vi "CRYAcquisition Editor.vi"() -> ()   [LabVIEW 2013]
uses:
  <vilib>/Utility/miscctls.llb/LVBoundsTypeDef.ctl
  Typedef Control/CRYAcquisition Cluster.ctl
  Typedef Control/CRYHardware Channel Info.ctl
  Typedef Control/CRYWaveform Cluster.ctl
  Typedef Control/CRYData Cluster.ctl
  CRYMainGlobal.vi
  CRYProject/CRYProject Editor Global.vi
  CRYWindow/SubVI/CRYMain Sub Window Global.vi
  Misc/SubVI/CRYMisc vis settings global.vi
  CRYStepSetup/CRYStepSetup Global.vi
panel:
  out "Acquisition Bk":T1={"Mode"=1, "Name"="", "use ch name"=FALSE, "Record Time"=10.0, "hide rec"=FALSE, "hide play"=FALSE, "rec delay"=0.0, "rec pad"=0.0, "dcc units"=0, "sine gen setting"="", "scope_fft setting"="", "voltmeter setting"="", "rta setting"="", "trig offset(sec)"=0.0, "triggered  record"=FALSE, "trig level"=0.0, "trig unit"=0, "trig slop"=FALSE, "trig timeout(sec)"=0.0, "add record"=FALSE, "EQ"=FALSE, "record table"=[], "play table"=[], "trig channel"="", "Help"=""} {"trig timeout(sec)" format="%.2f"; "trig level" format="%.2f"; "trig offset(sec)" format="%.2f"; "rec delay" format="%.2f"; "rec pad" format="%.2f"; "Record Time" format="%.2f"}
  out "Origin MR0":string[][](array[string])
  in  "Channels Change?":bool
  in  "Change Record Name?":bool
  out "Old MR0":string[][](array[string])
  out "Changed Curve":string[][](array[string])
  in  "AddStep":bool
  in  "Add Lib":bool
  in  "Board Tab":enum32{"Page 1"}(tab)
  in  "Cancel":bool caption="Apply"
  in  "OK":bool caption="Apply"
  in  "Sub Board Tab":enum32{"Setting", "Help"}(tab)
  in  "Mode Tab":T2(tab)
  out "Record0":bool caption="采集"
  in  "WFMRing":u16(ring) items=["Stimulus"]
  in  "MP0":i32(listbox)
  in  "O_Channel0":bool
  out "MR0":string[][](table)
  in  "I_Channel0":bool caption="Boolean 2"
  in  "Time R0":dbl caption="预采集时间(秒)" format="%#_6p"
  out "Play0":bool caption="播放"
  out "Trigger Boolean":bool caption="Record Trigger"
  in  "Triger1":bool caption="触发"
  in  "Trigger Level1":dbl caption="触发电平" format="%#.3p"
  in  "Trigger Offset1":dbl caption="触发偏移(s)" format="%#.3p"
  in  "Trigger Channel1":u16(ring) caption="触发通道" items=["Direct In 1", "Direct In 2", "Direct In 3", "Direct In 4", "Mic 1", "Mic 2", "Mic 3", "Mic 4", "DUT Mic L", "DUT Mic Current L", "Imp 1L", "Imp 1R", "LineIn L", "LineIn R", "USB In L", "USB In R"]
  in  "Time Out1":dbl caption="时间结束(s)" format="%#.3p"
  in  "Trigger Unit1_1":bool caption="触发单位"
  in  "Trigger Unit1_2":bool caption="Trigger Unit Pa"
  in  "Slop1+1":bool caption="斜率"
  in  "Slop1-1":bool
  in  "I_Channel1":bool
  in  "Time R1":dbl caption="采集时间(秒)" format="%#_6p"
  in  "MR1":string[][](table)
  out "Record1":bool caption="采集"
  out "Record1_1":bool caption="采集触发"
  in  "Hide P P2":bool caption="隐藏面板"
  in  "Config P2":bool
  out "Play2":bool caption="播放"
  in  "HideP R3":bool caption="隐藏面板"
  in  "Config R3":bool
  in  "MR3":string[][](table)
  out "Record3":bool caption="采集"
  in  "Config R4":bool
  in  "Hide P R4":bool caption="隐藏面板"
  in  "MR4":string[][](table)
  out "Record4":bool caption="采集"
  in  "Config R5":bool
  in  "Hide P R5":bool caption="隐藏面板"
  in  "MR5":string[][](table)
  out "Record5":bool caption="采集"
  in  "Config R6":bool
  in  "Hide P R6":bool caption="隐藏面板"
  in  "Delay R6":dbl caption="采集延迟(秒)" format="%#_6p"
  in  "MR6":string[][](table)
  out "Record6":bool caption="采集"
  in  "Hide P P7":bool caption="隐藏面板"
  in  "Config P7":bool
  in  "Config R7":bool
  in  "Hide P R7":bool caption="隐藏面板"
  in  "Delay R7":dbl caption="采集延迟(秒)" format="%#_6p"
  in  "MR7":string[][](table)
  out "Record7":bool caption="采集"
  out "Play7":bool caption="播放"
  in  "Hide P P8":bool caption="隐藏面板"
  in  "Config P8":bool
  in  "Config R8":bool
  in  "Hide P R8":bool caption="隐藏面板"
  in  "Delay R8":dbl caption="采集延迟(秒)" format="%#_6p"
  in  "MR8":string[][](table)
  out "Record8":bool caption="采集"
  out "Play8":bool caption="播放"
  in  "Hide P P9":bool caption="隐藏面板"
  in  "Config P9":bool
  in  "Config R9":bool
  in  "Hide P R9":bool caption="隐藏面板"
  in  "Delay R9":dbl caption="采集延迟(秒)" format="%#_6p"
  in  "MR9":string[][](table)
  out "Record9":bool caption="采集"
  out "Play9":bool caption="播放"
  in  "Hide P P10":bool caption="隐藏面板"
  in  "Config P10":bool
  in  "Config R10":bool
  in  "Hide P R10":bool caption="隐藏面板"
  in  "Delay R10":dbl caption="采集延迟(秒)" format="%#_6p"
  in  "MR10":string[][](table)
  out "Record10":bool caption="采集"
  out "Play10":bool caption="播放"
  in  "Record11":enum32{"Radio Selection 1", "Radio Selection 2"}(radio) caption="采集"
  out "Discription String":string
  in  "Record Curve Name":string caption="记录曲线名称"
  in  "Use Channel Name":bool=TRUE caption="使用通道名称"
  in  "Mode Select":u16(ring) caption="模式选择" items=["播放和采集", "采集", "信号发生器", "多功能表", "示波器", "频谱分析仪", "实时频谱分析仪", "信号发生器/多功能表", "信号发生器/示波器", "信号发生器/频谱分析仪", "信号发生器/实时频谱分析仪", "读取直流连接"]
  in  "Help":string
  in  "Apply":bool
  in  "Load...":bool caption="Apply"
  in  "Revert":bool caption="Apply"
  in  "Save As...":bool caption="Apply"
  in  "CurveReplace":bool caption="Use Channel Name"
  out "EndFlag":bool
  in  "Curve Change":enum16{"Curves", "Values", "Results", "WFM"}[](array[ring])
  in  "Started":bool
  in  "Execution control":T3={"interactive"=TRUE, "displayed"=TRUE, "in a seq"=FALSE}
  in  "Run flag":bool caption="Use Channel Name"
  out "Selected I_channel Info":T4[](array[typedef]) {"Coupling" items=["Default"=-1, "RSE"=10083, "NRSE"=10078, "Differential"=10106, "Pseudodifferential"=12529]; "term config" items=["Default"=-1, "RSE"=10083, "NRSE"=10078, "Differential"=10106, "Pseudodifferential"=12529]; "Anti-aliasing Factor (%fs)" format="%.2f"}
  out "Selected O_channel Info":T4[](array[typedef]) {"Coupling" items=["Default"=-1, "RSE"=10083, "NRSE"=10078, "Differential"=10106, "Pseudodifferential"=12529]; "term config" items=["Default"=-1, "RSE"=10083, "NRSE"=10078, "Differential"=10106, "Pseudodifferential"=12529]; "Anti-aliasing Factor (%fs)" format="%.2f"}
  in  "Calibration In":string
  in  "Hardware In":string
  in  "stop":bool
  out "Column":i32
  out "Row":i32
  out "I_channel Info":T4[](array[typedef]) caption="I_channel Info Out" {"Coupling" items=["Default"=-1, "RSE"=10083, "NRSE"=10078, "Differential"=10106, "Pseudodifferential"=12529]; "term config" items=["Default"=-1, "RSE"=10083, "NRSE"=10078, "Differential"=10106, "Pseudodifferential"=12529]; "Anti-aliasing Factor (%fs)" format="%.2f"}
  out "O_channel Info":T4[](array[typedef]) {"Coupling" items=["Default"=-1, "RSE"=10083, "NRSE"=10078, "Differential"=10106, "Pseudodifferential"=12529]; "term config" items=["Default"=-1, "RSE"=10083, "NRSE"=10078, "Differential"=10106, "Pseudodifferential"=12529]; "Anti-aliasing Factor (%fs)" format="%.2f"}
  out "Proper VI No":i32
  in  "Load Test":bool
  in  "Acquisition":T1={"Mode"=1, "Name"="", "use ch name"=FALSE, "Record Time"=10.0, "hide rec"=FALSE, "hide play"=FALSE, "rec delay"=0.0, "rec pad"=0.0, "dcc units"=0, "sine gen setting"="", "scope_fft setting"="", "voltmeter setting"="", "rta setting"="", "trig offset(sec)"=0.0, "triggered  record"=FALSE, "trig level"=0.0, "trig unit"=0, "trig slop"=FALSE, "trig timeout(sec)"=0.0, "add record"=FALSE, "EQ"=FALSE, "record table"=[], "play table"=[], "trig channel"="", "Help"=""} {"trig timeout(sec)" format="%.2f"; "trig level" format="%.2f"; "trig offset(sec)" format="%.2f"; "rec delay" format="%.2f"; "rec pad" format="%.2f"; "Record Time" format="%.2f"}
  out "VIMiniumBound":T5
  # "dB"
  # "+"
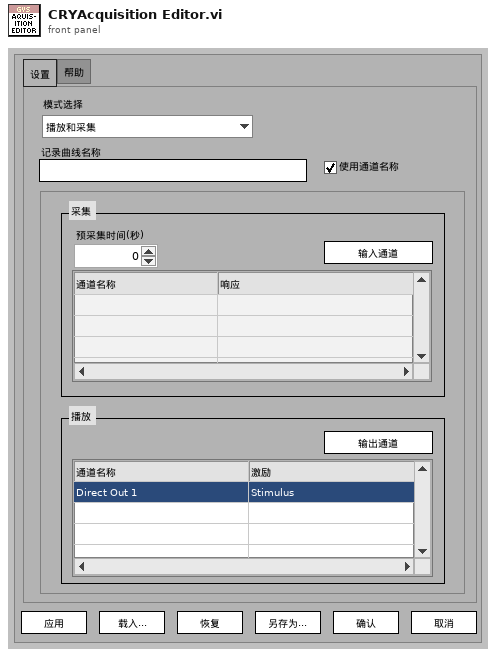
[diagram p1: front panel]
types:
  T1 = typedef "CRYAcquisition Cluster.ctl" = cluster{"Mode":u16, "Name":string, "use ch name":bool, "Record Time":dbl, "hide rec":bool, "hide play":bool, "rec delay":dbl, "rec pad":dbl, "dcc units":i8, "sine gen setting":string, "scope_fft setting":string, "voltmeter setting":string, "rta setting":string, "trig offset(sec)":dbl, "triggered  record":bool, "trig level":dbl, "trig unit":u8, "trig slop":bool, "trig timeout(sec)":dbl, "add record":bool, "EQ":bool, "record table":string[][], "play table":string[][], "trig channel":string, "Help":string}
  T2 = enum32{"0", "1", "2", "3", "4", "5", "6", "7", "8", "9", "10", "11"}
  T3 = cluster{"interactive":bool, "displayed":bool, "in a seq":bool}
  T4 = typedef "CRYHardware Channel Info.ctl" = cluster{"ID":i32, "Name":string, "Digital":bool, "Input":bool, "Device Name":string, "Hardware Ch ID":u8, "Vmax (V)":dbl, "Latency (samples)":dbl, "Sampling Rate (Hz)":u32, "Bit Depth":u32, "Anti-aliasing Factor (%fs)":sgl, "DAQmx Channel":tag, "term config":i32, "Coupling":i32, "IEPE en":bool, "ASIOChannel Name":string, "Audio Driver":u16, "ASIOChannel Index":u8}
  T5 = typedef "LVBoundsTypeDef.ctl" = cluster{"Width":u32, "Height":u32}
  T6 = typedef "CRYData Cluster.ctl" = cluster{"Name":string, "Curve":cluster{"x":dbl, "y":dbl, "z":dbl}[], "X data":u16, "Y data":u16, "Z data":u16, "X axis":u16, "Y axis":u16, "Z axis":u16, "X unit":string, "Y unit":string, "Z unit":string, "X dB ref":dbl, "Y dB ref":dbl, "Z dB ref":dbl, "single val":bool, "protected":bool, "display X":bool, "display Y":bool, "display Z":bool, "Test Info":string, "Step No.":i32, "Plot Settings":cluster{"Color":u32, "Interpolation":u8, "Point Style":u8, "Line Style":u8, "Point Color":u32, "Line Width":u8, "Bar Plot Style":u8, "Fill To":i16}, "AutoProtect":bool}
  T7 = typedef "CRYWaveform Cluster.ctl" = cluster{"Waveform":cluster{"X0":dbl, "dX":dbl, "Y":sgl[]}, "X data":u16, "Y data":u16, "Y axis":u16, "X unit":string, "Y unit":string, "Y dB ref":dbl, "display Y":bool, "display X":bool, "Overload?":bool, "Test Info":string, "Step No.":i32, "Name":string, "protected":bool, "Sqc history":string[], "Signal Channel ID":i32, "Plot Settings":cluster{"Color":u32, "Interpolation":u8, "Point Style":u8, "Line Style":u8, "Point Color":u32, "Line Width":u8, "Bar Plot Style":u8, "Fill To":i16}, "AutoProtect":bool}
  T8 = typedef "CRYStep.ctl" = cluster{"No.VI":i32, "Category":string, "StepName":string, "Seq setup flattened":string, "Comment":string, "Steps config.":bool[], "Jump config":i32[], "Start":dbl, "Increment":dbl, "Name":string, "Unit":string, "Y data":u16, "Y prefix":string, "Y dB ref":dbl, "Y unit":string, "Repeat State Array":cluster{"Start":dbl, "Increment":dbl, "Count":i32, "Num":i32}[]}
  T9 = enum16{"OK", "Yes", "YesNo", "YesNoCancel", "ReplaceAppend"}
  T10 = typedef "LVPoint32TypeDef.ctl" = cluster{"Horizontal":i32, "Vertical":i32}
  T11 = typedef "LVRowAndColumnTypeDef.ctl" = cluster{"Row":i32, "Column":i32}
  T12 = typedef "LVPositionTypeDef.ctl" = cluster{"Left":i32, "Top":i32}
  T13 = typedef "CRYWaveform Cluster Array.ctl" = T7[]
  T14 = typedef "CRYCalibration 2DCluster.ctl" = cluster{"Calibration":T15, "Corr Curve":T6, "EQ Curve":T6, "Sens Curve":T6}
  T15 = typedef "CRYCalibration Cluster.ctl" = cluster{"Calibration Step Name":string, "Device":string, "Correction Curve Name":string, "Equalization Curve Name":string, "Sensitivity Curve Name":string, "Corr Folder and File":string, "EQ Folder and File":string, "Sens Folder and File":string, "Corr Step size":u16, "EQ Step size":u16, "Input":bool, "Last Cal Date (sec)":timestamp, "Cha Name":string, "Corr Curve Found":bool, "EQ Curve Found":bool, "Sens Curve Found":bool, "Signal Type":string, "Calibrated Device":string, "Hz":u32}
  T16 = cluster{"Load Test":bool, "I_Channel0":bool, "O_Channel0":bool, "I_Channel1":bool, "Config P2":bool, "Config R3":bool, "Config R4":bool, "Config R5":bool, "Config R6":bool, "Config R7":bool, "Config P7":bool, "Config R8":bool, "Config P8":bool, "Config R9":bool, "Config P9":bool, "Config R10":bool, "Config P10":bool, "Add Lib":bool, "OK":bool, "Cancel":bool}
  T17 = typedef "CRYCalibration All Cluster.ctl" = cluster{"Calibration 2D":T14[], "Help":string, "Tab Value":i32, "Input Signal Type":string, "Output Signal Type":string}
  T18 = typedef "CRYHardware.ctl" = cluster{"Name":string, "Analog I/O":u16, "Digital I/O":u16, "Channels":u8, "Dig Dev ID":u8, "N ports":u8, "Interface":u32, "Dig I/O Ports":cluster{"port #":i16, "width":i16, "direction":i32}[], "Interf settings":cluster{"Type":u16, "COM Port":u8, "Baud rate":u32, "Data bits":u32, "Parity":u16, "Stop bits":u16, "Flow control":u16, "Dev ID IEEE":u8}[], "N interfs":i32, "udev SNs":i16[], "udev enable":bool, "Channel Array":T4[], "Cal sequence":string, "SelectedIn":u16, "SelectedOut":u16, "SelectedTab":u16, "State":bool, "Help":string, "Advanced":bool, "In Audio Driver":u16, "Out Audio Driver":u16}
  T19 = cluster{"StepName":string, "setup flattened":string}[]
  T20 = cluster{"StepName":string, "setup flattened":string}
  T21 = typedef "CRYStimulus Cluster.ctl" = cluster{"StimulusType":string, "UseMLValArray":u16[], "ML_axisArray":u16[], "MLValLevelNameArray":string[], "Level(U)Array":dbl[], "Start(Stop)FreqArray":dbl[], "Start(Stop)AmpArray":dbl[], "StepResolutionArray":u16[], "Unit_Array":u16[], "DegValArray":dbl[], "DegUnitArray":string[], "Steps1":i32, "Cycle/step1(#)":u32, "Time/step1(s)":dbl, "Transition1":dbl, "SweepRate2":dbl, "Freq3(Hz)":dbl, "Steps3(#)":dbl, "Cycles3(#)":u32, "StepSize3":dbl, "wave time":string, "RMS_Value4":dbl, "Peak_Value4":dbl, "WavePath4":string, "RMS_unit4":string, "Peak_unit4":string, "wave Info":string, "dc_ctrl5_1":u16, "dc_ctrl5_2":u16, "dc_polar5":u16, "Max.Current":u16, "Steps5(#)":u32, "Time/Step5":dbl, "Level5":dbl, "StepsSize5Val":dbl, "StepSize5Unit":string, "SweepType":u16, "Fixed/Ratio6":u16, "Transition6":dbl, "Steps6(#)":dbl, "Cycle/Steps6(#)":u32, "Time/Steps6(s)":dbl, "Freq6(Hz)":dbl, "Difference6(Hz)":dbl, "Ratio6":string, "NoiseType7":u16, "Duration7(s)":dbl, "MinFreq7(Hz)":dbl, "MaxFreq7(Hz)":dbl, "MinFreq8(Hz)":dbl, "MaxFreq8(Hz)":dbl, "FreqRounding8":bool, "Duration8(s)":dbl, "Tones8":dbl, "RoundingVal8":dbl, "ApplyEQ":bool, "Duration(s)":dbl, "CustomStimulusName ":string, "Flatten Element Array":string[], "sine waves":cluster{"freq":dbl, "ampl":dbl, "cycles":dbl}[], "Channel Out":i32, "RatioVal6":dbl, "TabCtrl6":enum32{"Master Tone", "Slave Tone"}, "Signal Type Name":string, "Help":string, "Channel Sel":u16, "V on DUT":bool, "Output Imp":dbl, "Nominal Imp":dbl}
  T22 = cluster{"Signal Type":string, "CustomStimulusName ":string}
  T23 = cluster{"gen'r mode":i32, "frequency":u32, "output level":dbl, "wave path":string, "wav play mode":i32, "duration":dbl, "n times":i32, "channel":i32, "wav level":dbl, "EQ":bool, "f knob log":bool, "f knob low":dbl, "f knob high":dbl, "ol knob log":bool, "ol knob low":dbl, "ol knob high":dbl, "Lin Display Prefs":string, "dB Display Prefs":string, "Duration noise":dbl, "Min freq noise":dbl, "Max freq noise":dbl, "Channel String":string, "Play Sine Wave":i32}
  T24 = typedef "CRYMultimeter.ctl" = cluster{"Ave/Max/Min":i32, "Level":i32, "Channel":i32, "Signal Type":string, "Weighting":string, "Applay Correction":bool, "lin/exp avg":u16, "rec time (sec)":dbl, "Average Time (Sec)":dbl, "Lin Display Prefs":string, "dB Display Prefs":string, "Time Weighting":u16, "Display":u16}
  T25 = typedef "CRYScope-FFT.ctl" = cluster{"window":i32, "n avgs":i32, "lin/exp avg":i32, "pwr/cplx avg":i32, "time (ms)":dbl, "fft lines":i32, "scope/fft mode":i32, "channel":i32, "trig. channel":i32, "Applay Correction":bool, "Time Display":string, "Freq. Weighting":string, "Ave/Max/Min":u16, "Trigger Level":dbl, "Trigger Unit":u16, "Trigger Time Offset":dbl, "Trigger Slope":u16, "Trigger/Free Run":bool, "continuous":bool, "Spectrum Display":string, "Calc FFT":bool, "Y-axis":string, "Signal Type":string}
  T26 = cluster{"octave":i32, "det time":i32, "det sec":dbl, "lin/exp":i32, "weighting":i32, "channel":i32, "Ave/Max/Min":u16, "continuous":bool, "Applay Correction":bool, "Display":u16, "Channel String":string}
  T27 = cluster{"octave":i32, "det time":i32, "det sec":dbl, "lin/exp":i32, "weighting":i32, "channel":i32, "Ave/Max/Min":u16, "continuous":bool, "Applay Correction":bool, "Display":u16, "Signal Type":string}
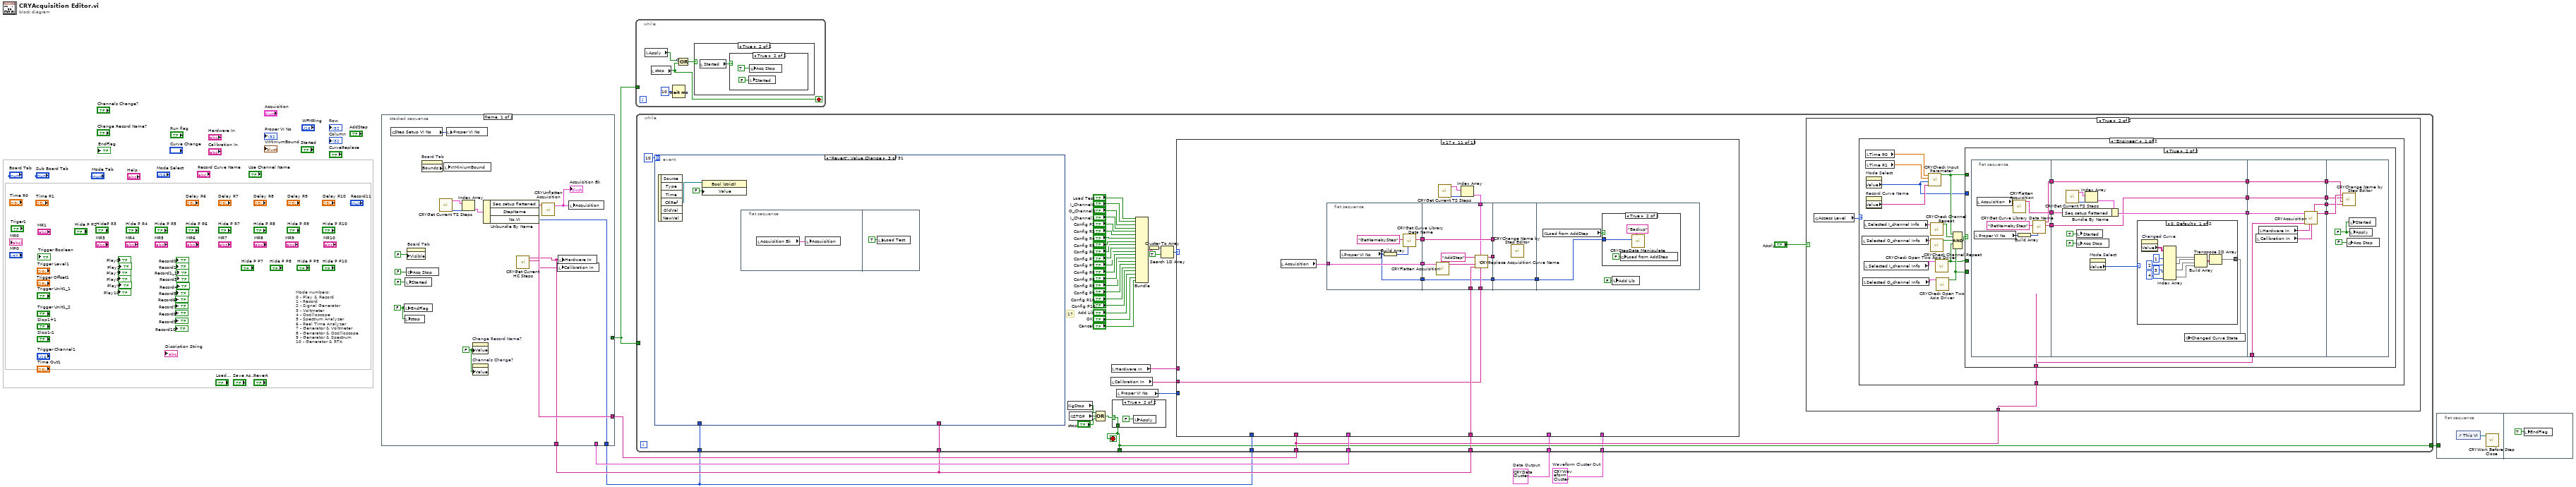
[diagram p0: block diagram]
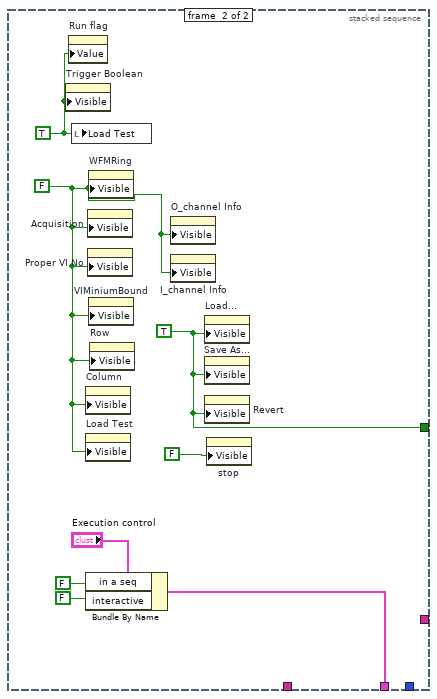
[diagram p4: hidden frame]
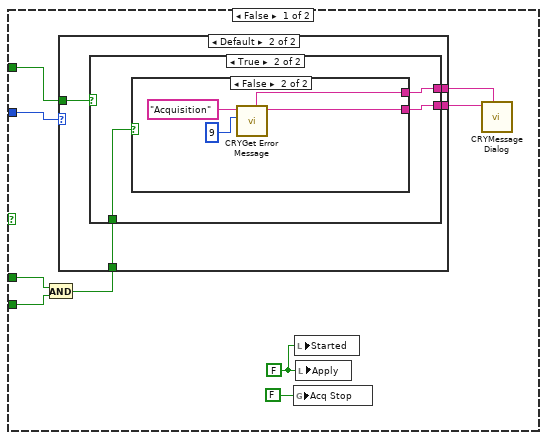
[diagram p7: hidden frame]
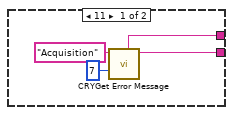
[diagram p8: hidden frame]
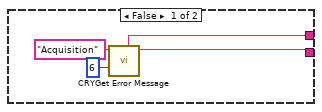
[diagram p9: hidden frame]
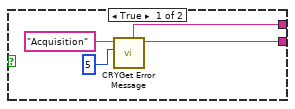
[diagram p10: hidden frame]
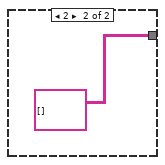
[diagram p11: hidden frame]
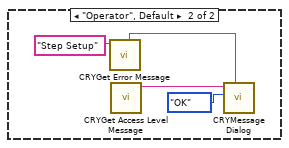
[diagram p12: hidden frame]
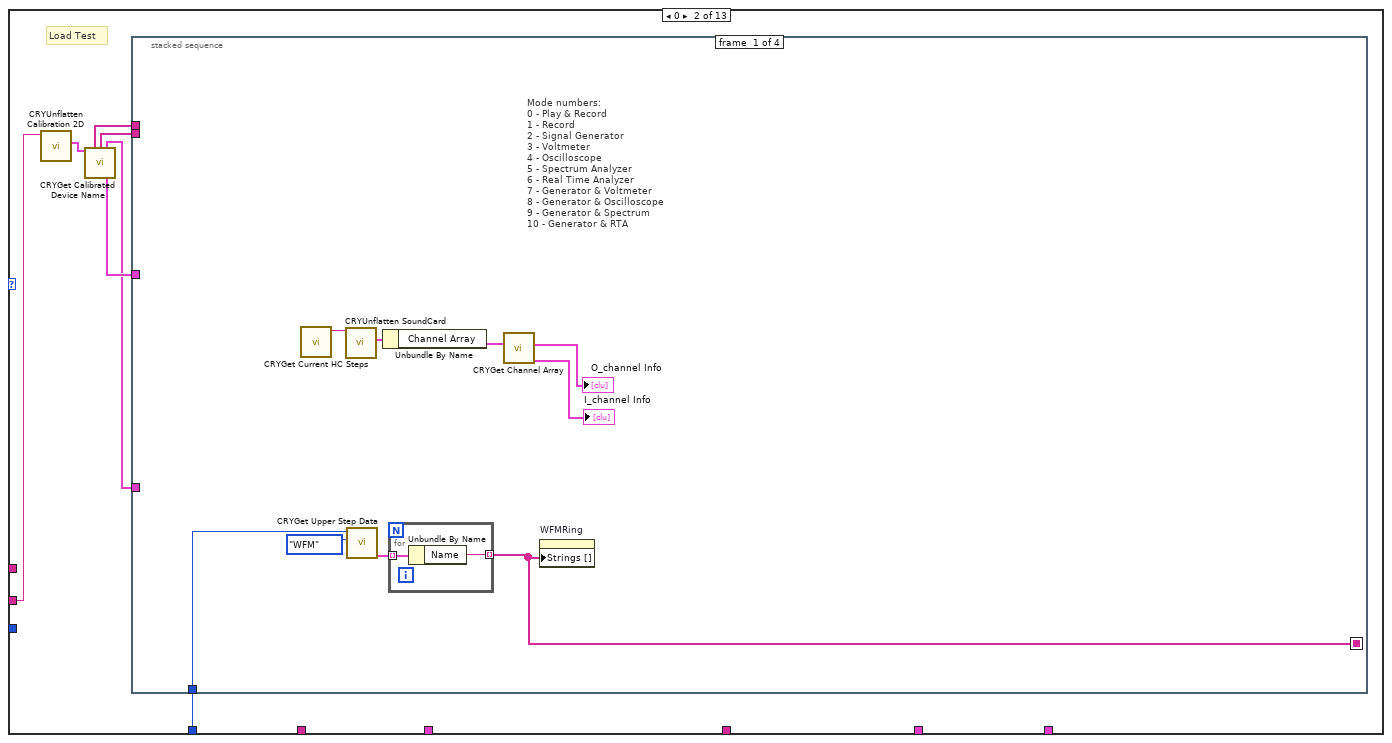
[diagram p14: hidden frame]
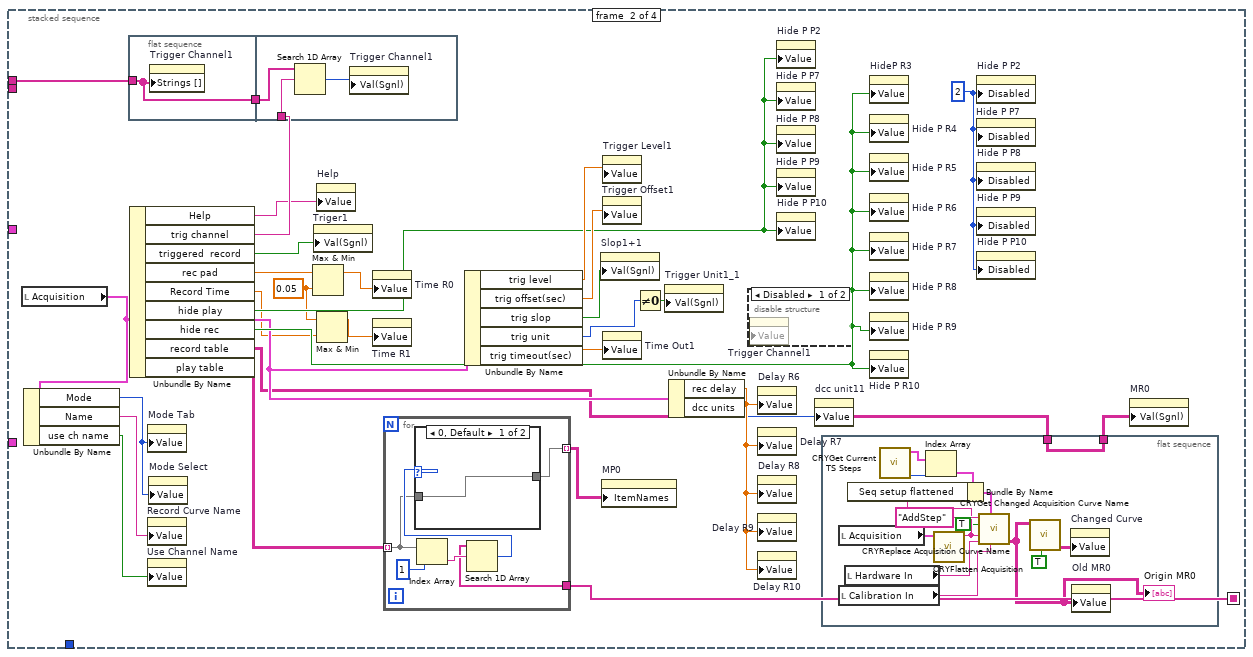
[diagram p15: hidden frame]
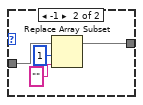
[diagram p16: hidden frame]
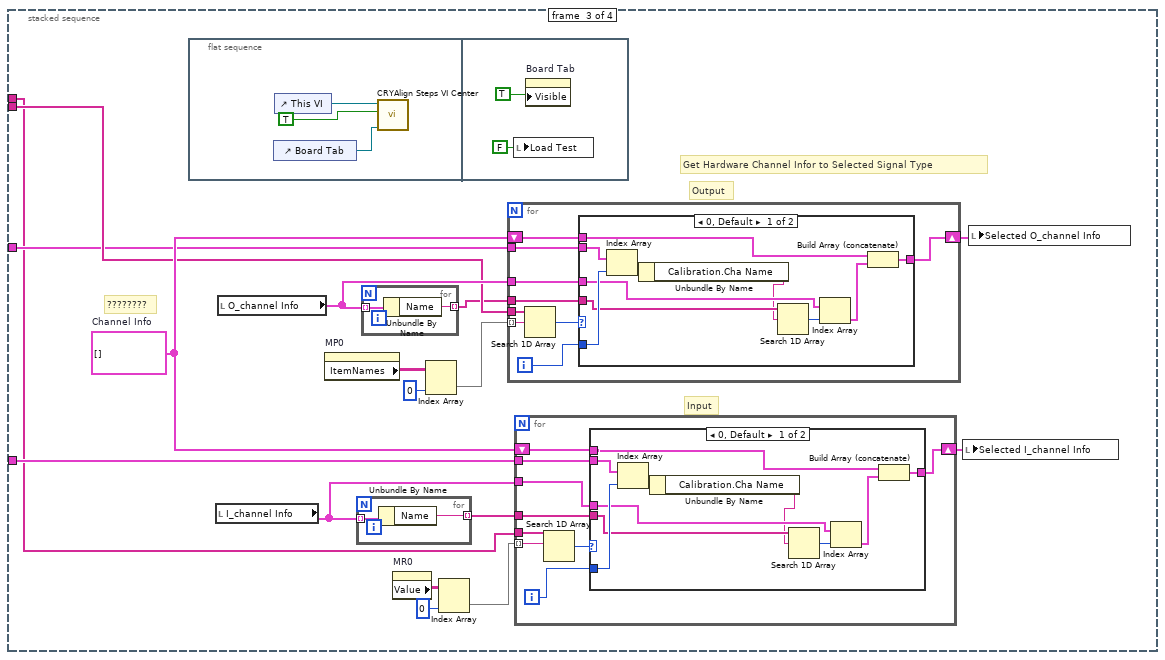
[diagram p18: hidden frame]
diagram:
  w5 = T6 {"Name"="", "Curve"=[], "X data"=1, "Y data"=1, "Z data"=1, "X axis"=0, "Y axis"=1, "Z axis"=1, "X unit"="Hz", "Y unit"="", "Z unit"="deg.", "X dB ref"=1.0, "Y dB ref"=1.0, "Z dB ref"=1.0, "single val"=FALSE, "protected"=FALSE, "display X"=TRUE, "display Y"=TRUE, "display Z"=TRUE, "Test Info"="", "Step No."=0, "Plot Settings"={"Color"=0, "Interpolation"=0, "Point Style"=0, "Line Style"=0, "Point Color"=0, "Line Width"=0, "Bar Plot Style"=0, "Fill To"=0}, "AutoProtect"=FALSE}  # Data Output
  w6 = T7 {"Waveform"={"X0"=0.0, "dX"=0.0, "Y"=[]}, "X data"=1, "Y data"=0, "Y axis"=0, "X unit"="s", "Y unit"="", "Y dB ref"=1.0, "display Y"=TRUE, "display X"=FALSE, "Overload?"=FALSE, "Test Info"="", "Step No."=0, "Name"="", "protected"=FALSE, "Sqc history"=[], "Signal Channel ID"=0, "Plot Settings"={"Color"=0, "Interpolation"=0, "Point Style"=0, "Line Style"=0, "Point Color"=0, "Line Width"=0, "Bar Plot Style"=0, "Fill To"=0}, "AutoProtect"=FALSE}  # Waveform Cluster Out
  # "Mode numbers:\n0 - Play & Record\n1 - Record\n2 - Signal Generator\n3 - Voltmeter\n4 - Oscilloscope\n5 - Spectrum Analyzer\n6 - Real Time Analyzer\n7 - Generator & Voltmeter\n8 - Generator & Oscilloscope\n9 - Generator & Spectrum\n10 - Generator & RTA"
  n1 = stacked-sequence {
    tunnel: [_ w25] -> w7
    tunnel: [w20 _] -> w4
    tunnel: [_ w27] -> w8
    tunnel: [w14 _] -> w3
    tunnel: [w11 _] -> w2
    frame #0 {
      w12 = FALSE ("Record Curve Name Change?")
      w9 = FALSE ("EndFlag")
      n2 = global read "CRYProject Editor Global.vi" "Step Setup VI No"() -> (w23:i32)
      n3 = local write "EndFlag"(w9) -> ()
      n4 = local write "stop"(w9) -> ()
      n5 = local write "Started"(FALSE ("Started")) -> ()
      n6 = global write "CRYMainGlobal.vi" "Acq Stop"(FALSE ("Acquisition Stop")) -> ()
      n7 = property on="Board Tab" class="TabCtl (strict)"("Visible"=FALSE) -> ()  [unwired: 2 in, 2 out]
      n8 = property on="Board Tab" class="TabCtl (strict)"() -> ("Bounds"=w15:T5)  [unwired: 2 in, 2 out]
      n9 = call "CRYGet Current TS Steps.vi"() -> ("SelectStepNumber in Tree"=w18:i32, "Steps"=w19:T8[])  [unwired: 1 in, 9 out]
      n10 = local write "VIMiniumBound"(w15) -> ()
      n11 = local write "Proper VI No"(w23) -> ()
      n12 = Index Array(array=w19, index=w18) -> (element=w21:T8)
      n13 = property on="Change Record Name?" class="Bool (strict)"("Value"=w12) -> ()  [unwired: 2 in, 2 out]
      n14 = property on="Channels Change?" class="Bool (strict)"("Value"=w12) -> ()  [unwired: 2 in, 2 out]
      n15 = Unbundle By Name(w21) -> ("Seq setup flattened"=w22:string, "StepName"=w20:string, "No.VI"=w11:i32)
      n16 = call "CRYGet Current HC Steps.vi"() -> ("Calibration setup flattened Out"=w13:string, "Hardware setup flattened Out"=w14:string)  [unwired: 10 in]
      n17 = call "CRYUnflatten Acquisition.vi"("Flatten Acquisition"=w22) -> ("Acquisition"=w10:T1)  [unwired: 10 out]
      "Acquisition Bk" <- w10
      n18 = local write "Calibration In"(w13) -> ()
      n19 = local write "Hardware In"(w14) -> ()
      n20 = local write "Acquisition"(w10) -> ()
    }
    frame #1 {
      w25 = TRUE ("Visible")
      w32 = FALSE ("Visible")
      w31 = TRUE ("Load Test")
      n21 = property on="Trigger Boolean" class="Bool (strict)"("Visible"=w31) -> ()  [unwired: 2 in, 2 out]
      n22 = property on="Run flag" class="Bool (strict)"("Value"=w31) -> ()  [unwired: 2 in, 2 out]
      n23 = local write "Load Test"(w31) -> ()
      n24 = property on="Column" class="DigNum (strict)"("Visible"=w32) -> ()  [unwired: 2 in, 2 out]
      n25 = property on="Load Test" class="Bool (strict)"("Visible"=w32) -> ()  [unwired: 2 in, 2 out]
      n26 = Bundle By Name(cluster="Execution control", "in a seq"=FALSE, "interactive"=FALSE) -> (w27:T3)
      n27 = property on="Acquisition" class="Clust (strict)"("Visible"=w32) -> ()  [unwired: 2 in, 2 out]
      n28 = property on="Proper VI No" class="DigNum (strict)"("Visible"=w32) -> ()  [unwired: 2 in, 2 out]
      n29 = property on="WFMRing" class="Ring (strict)"("Visible"=w32) -> ()  [unwired: 2 in, 2 out]
      n30 = property on="VIMiniumBound" class="Clust (strict)"("Visible"=w32) -> ()  [unwired: 2 in, 2 out]
      n31 = property on="Row" class="DigNum (strict)"("Visible"=w32) -> ()  [unwired: 2 in, 2 out]
      n32 = property on="O_channel Info" class="Arr (strict)"("Visible"=w32) -> ()  [unwired: 2 in, 2 out]
      n33 = property on="I_channel Info" class="Arr (strict)"("Visible"=w32) -> ()  [unwired: 2 in, 2 out]
      n34 = property on="Load..." class="Bool (strict)"("Visible"=w25) -> ()  [unwired: 2 in, 2 out]
      n35 = property on="Save As..." class="Bool (strict)"("Visible"=w25) -> ()  [unwired: 2 in, 2 out]
      n36 = property on="Revert" class="Bool (strict)"("Visible"=w25) -> ()  [unwired: 2 in, 2 out]
      n37 = property on="stop" class="Bool (strict)"("Visible"=FALSE) -> ()  [unwired: 2 in, 2 out]
    }
  }
  n38 = while {
    tunnel: w7 -> [_]
    stop <- w34 stop-if-true
    n39 = local read "Apply"() -> (w33:bool)
    n40 = local read "stop"() -> (w34:bool)
    n41 = Wait (ms)(milliseconds to wait=u32 10) -> ()  [unwired: 1 out]
    n42 = Compound Arithmetic op=OR(invert w33, w34) -> (w35:bool)
    n43 = case shown="True" w35 {
      frame False {
      }
      frame True {
        n44 = local read "Started"() -> (w37:bool)
        n45 = case shown="True" w37 {
          frame False {
          }
          frame True {
            n46 = local write "Started"(FALSE ("Started")) -> ()
            n47 = global write "CRYMainGlobal.vi" "Acq Stop"(TRUE ("Acquisition Stop")) -> ()
          }
        }
      }
    }
  }
  n48 = while {
    tunnel: w7 -> [_]
    tunnel: w4 -> [w56]
    tunnel: w8 -> [w57]
    tunnel: w6 -> [w52]
    tunnel: w5 -> [w50]
    tunnel: [w43] -> _
    tunnel: w3 -> [w48]
    tunnel: w3 -> [w46]
    tunnel: w2 -> [w45]
    tunnel: w2 -> [w44]
    tunnel: [w43] -> w1
    stop <- w43 stop-if-true
    # "17"
    n49 = event shown="[2] \"Revert\": Value Change" {
      selector: _ -> [_ _ _ _ _ _ _ _ _ _ _ _ _ _ _ _ _ _ _ _ _ _ _ _ _ _ _ _ _ _ _]
      dyn-events: _ -> [_ _ _ _ _ _ _ _ _ _ _ _ _ _ _ _ _ _ _ _ _ _ _ _ _ _ _ _ _ _ _]
      timeout: 10 -> [_ _ _ _ _ _ _ _ _ _ _ _ _ _ _ _ _ _ _ _ _ _ _ _ _ _ _ _ _ _ _]
      tunnel: w48 -> [_ _ _ _ _ _ _ _ _ _ _ _ _ _ _ _ _ _ _ _ _ _ _ _ _ _ _ _ _ _ _]
      tunnel: w44 -> [_ _ _ _ _ _ _ _ _ _ _ _ w802 _ _ _ _ _ _ _ _ _ _ _ _ _ _ _ _ _ _]
      event Timeout {
        n50 = event-data() -> ()  [unwired: 4 out]
      }
      event "Load...": Value Change {
        n51 = event-data() -> ("CtlRef"=w671:refnum<vi>)  [unwired: 6 out]
        n52 = local read "Load Test"() -> (w672:bool)
        n53 = case shown="False" w672 {
          frame True {
          }
          frame False {
            n54 = global read "CRYMainGlobal.vi" "Steps path"() -> (w678:path)
            n55 = local read "Proper VI No"() -> (w673:i32)
            n56 = Build Path(base path=w678, name or relative path="CRYAcquisition") -> (appended path=w677:path)
            n57 = call "CRYStep Read.vi"("Category Name"="Acquisition" ("Step File Name"), "Proper VI No"=w673, "Step File Path"=w677) -> ("status"=w676:bool, "selected path"=w674:path, "Flatten Step"=w675:string)  [unwired: 1 in, 3 out]
            n58 = case shown="True" w676 {
              tunnel: w675 -> [_ w682]
              tunnel: w674 -> [_ w681]
              tunnel: w673 -> [_ w683]
              frame False {
              }
              frame True {
                n59 = call "CRYUnflatten Acquisition.vi"("Flatten Acquisition"=w682) -> ("Error?"=w685:bool, "Acquisition"=w684:T1)  [unwired: 9 out]
                n60 = case shown="False" w685 {
                  tunnel: w684 -> [w689 _]
                  tunnel: w683 -> [w688 _]
                  tunnel: w682 -> [w687 _]
                  tunnel: w681 -> [w686 _]
                  frame False {
                    n61 = flat-sequence {
                      tunnel: w689 -> [w701]
                      tunnel: w688 -> [w698]
                      tunnel: w687 -> [w697]
                      tunnel: w686 -> [w691]
                      frame #0 {
                        n62 = local write "Acquisition"(w701) -> ()
                        n63 = Strip Path(path=w691) -> (name=w693:string)  [unwired: 1 out]
                        n64 = Reverse String(1:w693) -> (0:w694:string)
                        n65 = Match Pattern(string=w694, regular expression="[.]") -> (after substring=w695:string)  [unwired: 4 out]
                        n66 = Reverse String(1:w695) -> (0:w690:string)
                        n67 = call "CRYPreUpdate Sequence.vi"("EventName"="Load", "StepName Arg3"=w690, "Proper VI No"=w698, "Project View Step Name Identifier Arg1"="", "Step flattened Arg2"=w697, "AllChangeFlg"=TRUE ("Name/Identifier")) -> ()  [unwired: 10 in]
                      }
                      frame #1 {
                        n68 = local write "Load Test"(TRUE ("Load Test")) -> ()
                      }
                    }
                  }
                  frame True {
                  }
                }
              }
            }
          }
        }
        n69 = property class="Bool (strict)"(reference=w671, "Value"=FALSE) -> ()  [unwired: 1 in, 2 out]
      }
      event "Revert": Value Change {
        n70 = event-data() -> ("CtlRef"=w703:refnum<vi>)  [unwired: 6 out]
        n71 = property class="Bool (strict)"(reference=w703, "Value"=FALSE) -> ()  [unwired: 1 in, 2 out]
        n72 = flat-sequence {
          frame #0 {
            n73 = local read "Acquisition Bk"() -> (w705:T1)
            n74 = local write "Acquisition"(w705) -> ()
          }
          frame #1 {
            n75 = local write "Load Test"(TRUE ("Load Test")) -> ()
          }
        }
      }
      event "Save As...": Value Change {
        n76 = event-data() -> ("CtlRef"=w707:refnum<vi>)  [unwired: 6 out]
        n77 = property class="Bool (strict)"(reference=w707, "Value"=FALSE) -> ()  [unwired: 1 in, 2 out]
        n78 = local read "Acquisition"() -> (w709:T1)
        n79 = call "CRYFlatten Acquisition.vi"("Acquisition"=w709) -> ("Acquisition flattened"=w715:string)  [unwired: 10 out]
        n80 = global read "CRYMainGlobal.vi" "Steps path"() -> (w711:path)
        n81 = disable-structure shown="Disabled" {
          frame Disabled {
            n82 = Concatenate Strings("-" ("string"), "Left/Right" ("string")) -> ()  [unwired: 1 out]
          }
          frame Enabled {
          }
        }
        n83 = Build Path(base path=w711, name or relative path="CRYAcquisition") -> (appended path=w710:path)
        n84 = local read "Proper VI No"() -> (w717:i32)
        n85 = call "CRYStep Write.vi"("StepIdentifier"="", "Default"=FALSE, "Proper VI No"=w717, "Category Name"="Acquisition" ("Step File Name"), "Step File Path"=w710, "Step flattened"=w715, "Step File Name"="Acquisition") -> ()  [unwired: 1 in, 4 out]
      }
      event Pane Size {
        n86 = event-data() -> ()  [unwired: 7 out]
        n87 = control-ref of="Board Tab"() -> (w721:refnum<vi>)
        n88 = control-ref of="This VI"() -> (w722:refnum<vi>)
        n89 = call "CRYAlign Steps VI Center.vi"("Tab2"=w721, "Input/Output"=TRUE ("Preview"), "VIRef"=w722) -> ()  [unwired: 1 in, 8 out]
      }
      event Panel Close {
        n90 = event-data() -> ()  [unwired: 5 out]
        n91 = control-ref of="This VI"() -> (w725:refnum<vi>)
        n92 = local write "Cancel"(TRUE ("Cancel")) -> ()
        n93 = call "CRYWork Before Step Close.vi"("StepVI Ref"=w725) -> ()  [unwired: 11 in]
      }
      event "Mode Select": Value Change {
        n94 = event-data() -> ("NewVal"=w735:u16)  [unwired: 5 out]
        n95 = flat-sequence {
          tunnel: w735 -> [w738]
          tunnel: [w737] -> w726
          frame #0 {
            n96 = local read "Acquisition"() -> (w736:T1)
            n97 = Bundle By Name(cluster=w736, "Mode"=w738) -> (w737:T1)
            n98 = local write "Acquisition"(w737) -> ()
          }
        }
        n99 = Equal To 0?(x=w735) -> (x = 0?=w732:bool)
        n100 = Equal?(x=w735, y=1 ("index")) -> (x = y?=w733:bool)
        n101 = Or(x=w732, y=w733) -> (x .or. y?=w734:bool)
        n102 = property on="Mode Tab" class="TabCtl (strict)"("Value"=w735) -> ()  [unwired: 2 in, 2 out]
        n103 = property on="MR0" class="Tbl (strict)"() -> ("Value"=w727:string[][])  [unwired: 2 in, 2 out]
        n104 = case shown="False" w734 {
          tunnel: w726 -> [w739 _]
          frame False {
            n105 = disable-structure shown="Disabled" {
              disable-tunnel: w739 -> [w740 _]
              frame Disabled {
                n106 = property on="MR0" class="Tbl (strict)"() -> ("Value"=w744:string[][])  [unwired: 2 in, 2 out]
                n107 = Index Array(array=w744) -> (element=w743:string[])  [unwired: 2 in]
                n108 = Build Array(w743) -> (w742:string[][])
                n109 = Bundle By Name(cluster=w740, "record table"=w742) -> (w741:T1)
                n110 = local write "Acquisition"(w741) -> ()
                n111 = property on="MR0" class="Tbl (strict)"("Val(Sgnl)"=w742) -> ()  [unwired: 2 in, 2 out]
              }
              frame Enabled {
              }
            }
          }
          frame True {
          }
        }
        n112 = Index Array(array=w727) -> (element=w728:string[])  [unwired: 2 in]
        n113 = Build Array(w728) -> (w729:string[][])
        n114 = Bundle By Name(cluster=w726, "record table"=w729) -> (w730:T1)
        n115 = local write "Acquisition"(w730) -> ()
        n116 = property on="MR0" class="Tbl (strict)"("Val(Sgnl)"=w729) -> ()  [unwired: 2 in, 2 out]
      }
      event "Record Curve Name": Value Change {
        n117 = event-data() -> ("NewVal"=w750:string)  [unwired: 6 out]
        n118 = property on="MR0" class="Tbl (strict)"() -> ("Value"=w749:string[][])  [unwired: 2 in, 2 out]
        n119 = flat-sequence {
          tunnel: w746 -> [w751]
          tunnel: [w751] -> w745
          frame #0 {
            n120 = property on="Change Record Name?" class="Bool (strict)"("Value"=TRUE ("Record Curve Name Change?")) -> ()  [unwired: 2 in, 2 out]
          }
        }
        n121 = for {
          tunnel: w749 -> [w756] mode=indexing
          tunnel: w750 -> [w754]
          tunnel: [w753] -> w746 mode=indexing
          n122 = Replace Array Subset(array=w756, new element=w754, index=1) -> (w753:string[])
        }
        n123 = local read "Acquisition"() -> (w748:T1)
        n124 = Bundle By Name(cluster=w748, "Name"=w750, "record table"=w746) -> (w747:T1)
        n125 = property on="MR0" class="Tbl (strict)"("Val(Sgnl)"=w745) -> ()  [unwired: 2 in, 2 out]
        n126 = local write "Acquisition"(w747) -> ()
      }
      event "Use Channel Name": Value Change {
        n127 = event-data() -> ("NewVal"=w768:bool)  [unwired: 6 out]
        n128 = local read "Acquisition"() -> (w770:T1)
        n129 = Bundle By Name(cluster=w770, "use ch name"=w768) -> (w761:T1)
        n130 = local write "Acquisition"(w761) -> ()
        n131 = property on="Changed Curve" class="Arr (strict)"() -> ("Value"=w769:string[][])  [unwired: 2 in, 2 out]
        n132 = property on="Old MR0" class="Arr (strict)"() -> ("Value"=w766:string[][])  [unwired: 2 in, 2 out]
        n133 = property on="Origin MR0" class="Arr (strict)"() -> ("Value"=w758:string[][])  [unwired: 2 in, 2 out]
        n134 = local read "Calibration In"() -> (w765:string)
        n135 = local read "Hardware In"() -> (w764:string)
        n136 = call "CRYFlatten Acquisition.vi"("Acquisition"=w761) -> ("Acquisition flattened"=w763:string)  [unwired: 10 out]
        n137 = call "CRYReplace Acquisition Curve Name.vi"("Calibration in"=w765, "Hardware Setup In"=w764, "Step Setup In"=w763, "No Insert CurveLib?"=TRUE, "Type In"="AddStep") -> ("Current Name Out"=w760:string[][])  [unwired: 4 in, 2 out]
        n138 = call "CRYGet Changed Acquisition Curve Name.vi"("Change Record Curve Name?"=TRUE ("Record Curve Name Change?"), "Origin MR0"=w758, "Changed Name Table in"=w769, "use ch name"=w768, "Old Name"=w766, "New Name"=w760) -> ("Changed Name Table  out"=w759:string[][])  [unwired: 5 in]
        n139 = flat-sequence {
          tunnel: w760 -> [w772]
          tunnel: w759 -> [w771]
          frame #0 {
            n140 = property on="Old MR0" class="Arr (strict)"("Value"=w772) -> ()  [unwired: 2 in, 2 out]
            n141 = property on="Changed Curve" class="Arr (strict)"("Value"=w771) -> ()  [unwired: 2 in, 2 out]
          }
        }
      }
      event "Time R0": Value Change {
        n142 = event-data() -> ("NewVal"=w774:dbl)  [unwired: 6 out]
        n143 = Max & Min(x=w774, y=0.05) -> (max(x,y)=w773:dbl)  [unwired: 1 out]
        n144 = local read "Acquisition"() -> (w777:T1)
        n145 = Bundle By Name(cluster=w777, "rec pad"=w773) -> (w776:T1)
        n146 = property on="Time R0" class="DigNum (strict)"("Value"=w773) -> ()  [unwired: 2 in, 2 out]
        n147 = local write "Acquisition"(w776) -> ()
      }
      event "MR0": Value Change {
        n148 = event-data() -> ("NewVal"=w794:string[][])  [unwired: 6 out]
        n149 = property on="MR1" class="Tbl (strict)"("Value"=w794) -> ()  [unwired: 2 in, 2 out]
        n150 = property on="MR0" class="Tbl (strict)"("Value"=w794) -> ()  [unwired: 2 in, 2 out]
        n151 = property on="Origin MR0" class="Arr (strict)"() -> ("Value"=w782:string[][])  [unwired: 2 in, 2 out]
        n152 = property on="Channels Change?" class="Bool (strict)"() -> ("Value"=w789:bool)  [unwired: 2 in, 2 out]
        n153 = property on="Old MR0" class="Arr (strict)"() -> ("Value"=w795:string[][])  [unwired: 2 in, 2 out]
        n154 = property on="Change Record Name?" class="Bool (strict)"() -> ("Value"=w791:bool)  [unwired: 2 in, 2 out]
        n155 = property on="Changed Curve" class="Arr (strict)"() -> ("Value"=w792:string[][])  [unwired: 2 in, 2 out]
        n156 = property on="Use Channel Name" class="Bool (strict)"() -> ("Value"=w793:bool)  [unwired: 2 in, 2 out]
        n157 = property on="MR3" class="Tbl (strict)"("Value"=w794) -> ()  [unwired: 2 in, 2 out]
        n158 = property on="MR4" class="Tbl (strict)"("Value"=w794) -> ()  [unwired: 2 in, 2 out]
        n159 = property on="MR5" class="Tbl (strict)"("Value"=w794) -> ()  [unwired: 2 in, 2 out]
        n160 = property on="MR6" class="Tbl (strict)"("Value"=w794) -> ()  [unwired: 2 in, 2 out]
        n161 = property on="MR7" class="Tbl (strict)"("Value"=w794) -> ()  [unwired: 2 in, 2 out]
        n162 = property on="MR8" class="Tbl (strict)"("Value"=w794) -> ()  [unwired: 2 in, 2 out]
        n163 = property on="MR9" class="Tbl (strict)"("Value"=w794) -> ()  [unwired: 2 in, 2 out]
        n164 = property on="MR10" class="Tbl (strict)"("Value"=w794) -> ()  [unwired: 2 in, 2 out]
        n165 = local read "Acquisition"() -> (w796:T1)
        n166 = Bundle By Name(cluster=w796, "record table"=w794) -> (w784:T1)
        n167 = local read "Calibration In"() -> (w785:string)
        n168 = local read "Hardware In"() -> (w786:string)
        n169 = local write "Acquisition"(w784) -> ()
        n170 = call "CRYGet Current TS Steps.vi"() -> ("SelectStepNumber in Tree"=w780:i32, "Steps"=w781:T8[])  [unwired: 1 in, 9 out]
        n171 = call "CRYFlatten Acquisition.vi"("Acquisition"=w784) -> ("Acquisition flattened"=w787:string)  [unwired: 10 out]
        n172 = Index Array(array=w781, index=w780) -> (element=w779:T8)
        n173 = flat-sequence {
          tunnel: w790 -> [_]
          tunnel: w783 -> [w797]
          frame #0 {
            w798 = FALSE ("Record Curve Name Change?")
            n174 = property on="Change Record Name?" class="Bool (strict)"("Value"=w798) -> ()  [unwired: 2 in, 2 out]
            n175 = property on="Channels Change?" class="Bool (strict)"("Value"=w798) -> ()  [unwired: 2 in, 2 out]
            "Old MR0" <- w797
          }
        }
        n176 = call "CRYReplace Acquisition Curve Name.vi"("Calibration in"=w785, "Setup in"=w779, "Hardware Setup In"=w786, "Step Setup In"=w787, "No Insert CurveLib?"=TRUE, "Type In"="AddStep") -> ("Current Name Out"=w783:string[][])  [unwired: 3 in, 2 out]
        n177 = call "CRYGet Changed Acquisition Curve Name.vi"("Change Record Curve Name?"=w791, "Origin MR0"=w782, "Change Channels"=w789, "Changed Name Table in"=w792, "use ch name"=w793, "Old Name"=w795, "New Name"=w783) -> ("Changed Name Table  out"=w790:string[][])  [unwired: 4 in]
        "Changed Curve" <- w790
      }
      event "MP0": Value Change {
        n178 = event-data() -> ()  [unwired: 7 out]
        n179 = property on="MP0" class="MCListbox (strict)"() -> ("ItemNames"=w800:string[][])  [unwired: 2 in, 2 out]
        n180 = local read "Acquisition"() -> (w801:T1)
        n181 = Bundle By Name(cluster=w801, "play table"=w800) -> (w799:T1)
        n182 = local write "Acquisition"(w799) -> ()
      }
      event "MP0": Mouse Down {
        n183 = event-data() -> ("Coords"=w814:T10)  [unwired: 8 out]
        n184 = invoke on="MP0" class="MCListbox (strict)" method="Point To Row Column"("Point"=w814) -> ("CellPosition"=w816:T11)  [unwired: 6 in, 6 out]
        n185 = property on="MP0" class="MCListbox (strict)"("ActiveCell"=w816) -> ("CellSize"=w812:T5, "ActiveCellPos"=w813:T12, "ItemNames"=w815:string[][])  [unwired: 2 in, 2 out]
        n186 = Unbundle By Name(w816) -> ("Row"=w806:i32, "Column"=w805:i32)
        n187 = Equal To 0?(x=w805) -> (x = 0?=w823:bool)
        n188 = Equal To 0?(x=w806) -> (x = 0?=w824:bool)
        n189 = Compound Arithmetic op=AND(w823, w824) -> (w822:bool)
        n190 = Array Size(array=w815) -> (size(s)=w825:i32[])
        n191 = Unbundle By Name(w813) -> ("Left"=w819:i32, "Top"=w818:i32)
        n192 = Index Array(array=w825, index=0) -> (element=w809:i32)
        n193 = Greater Or Equal To 0?(x=w806) -> (x >= 0?=w810:bool)
        n194 = Less?(x=w806, y=w809) -> (x < y?=w811:bool)
        n195 = Equal?(x=w805, y=1) -> (x = y?=w803:bool)
        n196 = Subtract(x=w818, y=3) -> (x-y=w820:i32)
        n197 = case shown="True" w822 {
          tunnel: w813 -> [_ w841]
          tunnel: w814 -> [_ w842]
          tunnel: w812 -> [_ w840]
          tunnel: [TRUE w828] -> w808
          frame False {
          }
          frame True {
            n198 = Unbundle By Name(w842) -> ("Horizontal"=w833:i32, "Vertical"=w837:i32)
            n199 = Unbundle By Name(w840) -> ("Width"=w839:u32, "Height"=w838:u32)
            n200 = Unbundle By Name(w841) -> ("Left"=w831:i32, "Top"=w829:i32)
            n201 = Add(x=w831, y=w839) -> (x+y=w832:u32)
            n202 = Add(x=w829, y=w838) -> (x+y=w830:u32)
            n203 = In Range and Coerce(upper limit=w832, x=w833, lower limit=w831) -> (In Range?=w836:bool)  [unwired: 1 out]
            n204 = In Range and Coerce(upper limit=w830, x=w837, lower limit=w829) -> (In Range?=w835:bool)  [unwired: 1 out]
            n205 = Compound Arithmetic op=AND(w836, w835) -> (w834:bool)
            n206 = case shown="False" w834 {
              tunnel: [FALSE TRUE] -> w828
              frame False {
              }
              frame True {
              }
            }
          }
        }
        n207 = Compound Arithmetic op=AND(w810, w811, w808, w803) -> (w807:bool)
        n208 = case shown="True" w807 {
          tunnel: w802 -> [_ w846]
          frame False {
            n209 = property on="WFMRing" class="Ring (strict)"("Visible"=FALSE) -> ()  [unwired: 2 in, 2 out]
          }
          frame True {
            n210 = flat-sequence {
              tunnel: [w849] -> w847
              tunnel: w846 -> [w848]
              tunnel: w847 -> [w854]
              frame #0 {
                n211 = call "CRYGet Upper Step Data.vi"("Type In"=enum16{"Curves", "Values", "Results", "WFM"}."WFM", "No.VI"=w848) -> ("Waveform Array"=w851:T13)  [unwired: 9 out]
                n212 = for {
                  tunnel: w851 -> [w853] mode=indexing
                  tunnel: [w852] -> w849 mode=indexing
                  n213 = Unbundle By Name(w853) -> ("Name"=w852:string)
                }
                n214 = property on="WFMRing" class="Ring (strict)"("Strings []"=w849) -> ()  [unwired: 2 in, 2 out]
              }
              frame #1 {
                n215 = property on="MP0" class="MCListbox (strict)"() -> ("ItemNames"=w862:string[][])  [unwired: 2 in, 2 out]
                n216 = local read "Row"() -> (w861:i32)
                n217 = Index Array(array=w862, index (row)=w861, index (col)=1 ("disabled index (col)")) -> (element=w859:string)
                n218 = Search 1D Array(1D array=w854, element=w859) -> (index of element=w856:i32)  [unwired: 1 out]
                n219 = Less Than 0?(x=w856) -> (x < 0?=w858:bool)
                n220 = Select(t=0, s=w858, f=w856) -> (s? t:f=w857:i32)
                n221 = property on="WFMRing" class="Ring (strict)"("Value"=w857) -> ()  [unwired: 2 in, 2 out]
              }
              frame #2 {
                n222 = property on="WFMRing" class="Ring (strict)"("Visible"=TRUE) -> ()  [unwired: 2 in, 2 out]
              }
            }
          }
        }
        n223 = Bundle("Left"=w819, w820) -> (w821:cluster{"Left":i32, i32})  [unwired: 1 out]
        n224 = property on="WFMRing" class="Ring (strict)"("Position"=w821, "NmdNumSize"=w812) -> ()  [unwired: 2 in, 2 out]
        n225 = local write "Column"(w805) -> ()
        n226 = local write "Row"(w806) -> ()
      }
      event "MP0": Mouse Move {
        n227 = event-data() -> ("Coords"=w866:T10)  [unwired: 5 out]
        n228 = invoke on="MP0" class="MCListbox (strict)" method="Point To Row Column"("Point"=w866) -> ("CellPosition"=w865:T11)  [unwired: 6 in, 6 out]
        n229 = Unbundle By Name(w865) -> ("Row"=w869:i32, "Column"=w867:i32)
        n230 = local read "Column"() -> (w868:i32)
        n231 = local read "Row"() -> (w870:i32)
        n232 = Not Equal?(x=w867, y=w868) -> (x != y?=w872:bool)
        n233 = Not Equal?(x=w869, y=w870) -> (x != y?=w871:bool)
        n234 = Or(x=w871, y=w872) -> (x .or. y?=w864:bool)
        n235 = case shown="True" w864 {
          frame False {
          }
          frame True {
            n236 = property on="WFMRing" class="Ring (strict)"("Visible"=FALSE) -> ()  [unwired: 2 in, 2 out]
          }
        }
      }
      event "WFMRing": Value Change {
        n237 = event-data() -> ()  [unwired: 7 out]
        n238 = property on="WFMRing" class="Ring (strict)"() -> ("RingText.Text"=w877:string)  [unwired: 2 in, 2 out]
        n239 = property on="MP0" class="MCListbox (strict)"() -> ("ItemNames"=w880:string[][])  [unwired: 2 in, 2 out]
        n240 = local read "Row"() -> (w879:i32)
        n241 = Replace Array Subset(array=w880, new element=w877, index (row)=w879, index (col)=1 ("disabled index (col)")) -> (w875:string[][])
        n242 = property on="MP0" class="MCListbox (strict)"("ItemNames"=w875) -> ()  [unwired: 2 in, 2 out]
        n243 = local read "Acquisition"() -> (w876:T1)
        n244 = Bundle By Name(cluster=w876, "play table"=w875) -> (w874:T1)
        n245 = local write "Acquisition"(w874) -> ()
      }
      event "WFMRing": Mouse Down {
        n246 = event-data() -> ()  [unwired: 9 out]
        n247 = property on="WFMRing" class="Ring (strict)"() -> ("RingText.Text"=w884:string)  [unwired: 2 in, 2 out]
        n248 = property on="MP0" class="MCListbox (strict)"() -> ("ItemNames"=w887:string[][])  [unwired: 2 in, 2 out]
        n249 = local read "Row"() -> (w886:i32)
        n250 = Replace Array Subset(array=w887, new element=w884, index (row)=w886, index (col)=1 ("disabled index (col)")) -> (w882:string[][])
        n251 = property on="MP0" class="MCListbox (strict)"("ItemNames"=w882) -> ()  [unwired: 2 in, 2 out]
        n252 = local read "Acquisition"() -> (w883:T1)
        n253 = Bundle By Name(cluster=w883, "play table"=w882) -> (w881:T1)
        n254 = local write "Acquisition"(w881) -> ()
      }
      event "Triger1": Value Change {
        n255 = event-data() -> ("NewVal"=w892:bool)  [unwired: 6 out]
        n256 = Not(x=w892) -> (.not. x?=w891:bool)
        n257 = property on="Trigger Boolean" class="Bool (strict)"("Visible"=w891) -> (error out=w888:errorcluster)  [unwired: 2 in, 1 out]
        n258 = local read "Load Test"() -> (w890:bool)
        n259 = property on="Trigger Channel1" class="Ring (strict)"(error in=w888) -> ("Value"=w889:u16)  [unwired: 1 in, 2 out]
        n260 = case shown="False" w890 {
          tunnel: w892 -> [w894 _]
          frame False {
            n261 = local read "Acquisition"() -> (w895:T1)
            n262 = Bundle By Name(cluster=w895, "triggered  record"=w894) -> (w893:T1)
            n263 = local write "Acquisition"(w893) -> ()
          }
          frame True {
          }
        }
        n264 = property on="Trigger Channel1" class="Ring (strict)"("Val(Sgnl)"=w889) -> ()  [unwired: 2 in, 2 out]
      }
      event "Trigger Level1": Value Change {
        n265 = event-data() -> ("NewVal"=w897:dbl)  [unwired: 6 out]
        n266 = local read "Acquisition"() -> (w898:T1)
        n267 = Bundle By Name(cluster=w898, "trig level"=w897) -> (w896:T1)
        n268 = local write "Acquisition"(w896) -> ()
      }
      event "Trigger Channel1": Value Change {
        n269 = event-data() -> ()  [unwired: 7 out]
        n270 = property on="Trigger Channel1" class="Ring (strict)"() -> ("RingText.Text"=w900:string)  [unwired: 2 in, 2 out]
        n271 = local read "Load Test"() -> (w899:bool)
        n272 = call "CRYGet Current Calibration Info.vi"("Is Input?"=TRUE, "Signal Type Name"=w900) -> ("Calibration All Cluster"=w910:T14)  [unwired: 9 in]
        n273 = case shown="False" w899 {
          tunnel: w900 -> [w913 _]
          frame False {
            n274 = local read "Acquisition"() -> (w914:T1)
            n275 = Bundle By Name(cluster=w914, "trig channel"=w913) -> (w912:T1)
            n276 = local write "Acquisition"(w912) -> ()
          }
          frame True {
          }
        }
        n277 = Unbundle By Name(w910) -> ("Sens Curve.Y unit"=w906:string)
        n278 = Search/Split String(string=w906, search string/char (-)="/" ("search char (-)")) -> (substring before match=w903:string, match + rest of string=w902:string, offset of match=w908:i32)  [unwired: 1 out]
        n279 = Greater Or Equal To 0?(x=w908) -> (x >= 0?=w907:bool)
        n280 = String Subset(string=w902, offset (0)=1) -> (substring=w901:string)  [unwired: 1 in]
        n281 = Select(t=w901, s=w907, f=w903) -> (s? t:f=w905:string)
        n282 = property on="Trigger Unit1_2" class="Bool (strict)"("BoolText.Text"=w905) -> ()  [unwired: 2 in, 2 out]
      }
      event "Trigger Offset1": Value Change {
        n283 = event-data() -> ("NewVal"=w916:dbl)  [unwired: 6 out]
        n284 = local read "Acquisition"() -> (w917:T1)
        n285 = Bundle By Name(cluster=w917, "trig offset(sec)"=w916) -> (w915:T1)
        n286 = local write "Acquisition"(w915) -> ()
      }
      event "Time Out1": Value Change {
        n287 = event-data() -> ("NewVal"=w919:dbl)  [unwired: 6 out]
        n288 = local read "Acquisition"() -> (w920:T1)
        n289 = Bundle By Name(cluster=w920, "trig timeout(sec)"=w919) -> (w918:T1)
        n290 = local write "Acquisition"(w918) -> ()
      }
      event "Time R1": Value Change {
        n291 = event-data() -> ("NewVal"=w922:dbl)  [unwired: 6 out]
        n292 = Max & Min(x=w922, y=0.05) -> (max(x,y)=w921:dbl)  [unwired: 1 out]
        n293 = property on="Time R1" class="DigNum (strict)"("Value"=w921) -> ()  [unwired: 2 in, 2 out]
        n294 = local read "Acquisition"() -> (w925:T1)
        n295 = Bundle By Name(cluster=w925, "Record Time"=w921) -> (w924:T1)
        n296 = local write "Acquisition"(w924) -> ()
      }
      event "Trigger Unit1_1": Value Change {
        n297 = event-data() -> ("NewVal"=w927:bool)  [unwired: 6 out]
        n298 = Not(x=w927) -> (.not. x?=w928:bool)
        n299 = property on="Trigger Unit1_1" class="Bool (strict)"("Value"=w927) -> ()  [unwired: 2 in, 2 out]
        n300 = property on="Trigger Unit1_2" class="Bool (strict)"("Value"=w928) -> ()  [unwired: 2 in, 2 out]
        n301 = local read "Load Test"() -> (w926:bool)
        n302 = case shown="False" w926 {
          tunnel: w927 -> [w931 _]
          frame False {
            n303 = Boolean To (0,1)(Boolean=w931) -> (0, 1=w930:i16)
            n304 = local read "Acquisition"() -> (w932:T1)
            n305 = Bundle By Name(cluster=w932, "trig unit"=w930) -> (w929:T1)
            n306 = local write "Acquisition"(w929) -> ()
          }
          frame True {
          }
        }
      }
      event "Trigger Unit1_2": Value Change {
        n307 = event-data() -> ("NewVal"=w937:bool)  [unwired: 6 out]
        n308 = Not(x=w937) -> (.not. x?=w934:bool)
        n309 = property on="Trigger Unit1_1" class="Bool (strict)"("Value"=w934) -> ()  [unwired: 2 in, 2 out]
        n310 = property on="Trigger Unit1_2" class="Bool (strict)"("Value"=w937) -> ()  [unwired: 2 in, 2 out]
        n311 = Boolean To (0,1)(Boolean=w934) -> (0, 1=w935:i16)
        n312 = local read "Acquisition"() -> (w936:T1)
        n313 = Bundle By Name(cluster=w936, "trig unit"=w935) -> (w933:T1)
        n314 = local write "Acquisition"(w933) -> ()
      }
      event "Slop1+1": Value Change {
        n315 = event-data() -> ("NewVal"=w939:bool)  [unwired: 6 out]
        n316 = Not(x=w939) -> (.not. x?=w940:bool)
        n317 = property on="Slop1+1" class="Bool (strict)"("Value"=w939) -> ()  [unwired: 2 in, 2 out]
        n318 = property on="Slop1-1" class="Bool (strict)"("Value"=w940) -> ()  [unwired: 2 in, 2 out]
        n319 = local read "Load Test"() -> (w938:bool)
        n320 = case shown="False" w938 {
          tunnel: w939 -> [w942 _]
          frame False {
            n321 = local read "Acquisition"() -> (w943:T1)
            n322 = Bundle By Name(cluster=w943, "trig slop"=w942) -> (w941:T1)
            n323 = local write "Acquisition"(w941) -> ()
          }
          frame True {
          }
        }
      }
      event "Slop1-1": Value Change {
        n324 = event-data() -> ("NewVal"=w947:bool)  [unwired: 6 out]
        n325 = Not(x=w947) -> (.not. x?=w945:bool)
        n326 = property on="Slop1+1" class="Bool (strict)"("Value"=w945) -> ()  [unwired: 2 in, 2 out]
        n327 = property on="Slop1-1" class="Bool (strict)"("Value"=w947) -> ()  [unwired: 2 in, 2 out]
        n328 = local read "Acquisition"() -> (w946:T1)
        n329 = Bundle By Name(cluster=w946, "trig slop"=w945) -> (w944:T1)
        n330 = local write "Acquisition"(w944) -> ()
      }
      event "Delay R6", "Delay R7", "Delay R8", "Delay R9", "Delay R10": Value Change {
        n331 = event-data() -> ("NewVal"=w949:dbl)  [unwired: 6 out]
        n332 = local read "Acquisition"() -> (w950:T1)
        n333 = property on="Delay R6" class="DigNum (strict)"("Value"=w949) -> ()  [unwired: 2 in, 2 out]
        n334 = property on="Delay R7" class="DigNum (strict)"("Value"=w949) -> ()  [unwired: 2 in, 2 out]
        n335 = property on="Delay R8" class="DigNum (strict)"("Value"=w949) -> ()  [unwired: 2 in, 2 out]
        n336 = property on="Delay R9" class="DigNum (strict)"("Value"=w949) -> ()  [unwired: 2 in, 2 out]
        n337 = property on="Delay R10" class="DigNum (strict)"("Value"=w949) -> ()  [unwired: 2 in, 2 out]
        n338 = Bundle By Name(cluster=w950, "rec delay"=w949) -> (w948:T1)
        n339 = local write "Acquisition"(w948) -> ()
      }
      event "HideP R3", "Hide P R4", "Hide P R5", "Hide P R7", "Hide P R8", "Hide P R9", "Hide P R10", "Hide P R6": Value Change {
        n340 = event-data() -> ("NewVal"=w952:bool)  [unwired: 6 out]
        n341 = local read "Acquisition"() -> (w953:T1)
        n342 = Bundle By Name(cluster=w953, "hide rec"=w952) -> (w951:T1)
        n343 = property on="HideP R3" class="Bool (strict)"("Value"=w952) -> ()  [unwired: 2 in, 2 out]
        n344 = property on="Hide P R4" class="Bool (strict)"("Value"=w952) -> ()  [unwired: 2 in, 2 out]
        n345 = property on="Hide P R5" class="Bool (strict)"("Value"=w952) -> ()  [unwired: 2 in, 2 out]
        n346 = property on="Hide P R6" class="Bool (strict)"("Value"=w952) -> ()  [unwired: 2 in, 2 out]
        n347 = property on="Hide P R7" class="Bool (strict)"("Value"=w952) -> ()  [unwired: 2 in, 2 out]
        n348 = property on="Hide P R8" class="Bool (strict)"("Value"=w952) -> ()  [unwired: 2 in, 2 out]
        n349 = property on="Hide P R9" class="Bool (strict)"("Value"=w952) -> ()  [unwired: 2 in, 2 out]
        n350 = property on="Hide P R10" class="Bool (strict)"("Value"=w952) -> ()  [unwired: 2 in, 2 out]
        n351 = local write "Acquisition"(w951) -> ()
      }
      event "Hide P P2", "Hide P P7", "Hide P P8", "Hide P P9", "Hide P P10": Value Change {
        n352 = event-data() -> ("NewVal"=w955:bool)  [unwired: 6 out]
        n353 = local read "Acquisition"() -> (w956:T1)
        n354 = Bundle By Name(cluster=w956, "hide play"=w955) -> (w954:T1)
        n355 = property on="Hide P P2" class="Bool (strict)"("Value"=w955) -> ()  [unwired: 2 in, 2 out]
        n356 = property on="Hide P P7" class="Bool (strict)"("Value"=w955) -> ()  [unwired: 2 in, 2 out]
        n357 = property on="Hide P P8" class="Bool (strict)"("Value"=w955) -> ()  [unwired: 2 in, 2 out]
        n358 = property on="Hide P P9" class="Bool (strict)"("Value"=w955) -> ()  [unwired: 2 in, 2 out]
        n359 = property on="Hide P P10" class="Bool (strict)"("Value"=w955) -> ()  [unwired: 2 in, 2 out]
        n360 = local write "Acquisition"(w954) -> ()
      }
      event "Record11": Value Change {
        n361 = event-data() -> ("NewVal"=w958:enum32{"Radio Selection 1", "Radio Selection 2"})  [unwired: 6 out]
        n362 = local read "Acquisition"() -> (w959:T1)
        n363 = Bundle By Name(cluster=w959, "dcc units"=w958) -> (w957:T1)
        n364 = local write "Acquisition"(w957) -> ()
      }
      event "Help": Value Change {
        n365 = event-data() -> ("NewVal"=w961:string)  [unwired: 6 out]
        n366 = local read "Acquisition"() -> (w962:T1)
        n367 = Bundle By Name(cluster=w962, "Help"=w961) -> (w960:T1)
        n368 = local write "Acquisition"(w960) -> ()
      }
    }
    n369 = global read "CRYMain Sub Window Global.vi" "gStop"() -> (w49:bool)
    n370 = global read "CRYMainGlobal.vi" "STOP"() -> (w55:bool)
    n371 = Compound Arithmetic op=OR(w49, w55, "stop") -> (w53:bool)
    n372 = local read "Calibration In"() -> (w58:string)
    n373 = local read "Hardware In"() -> (w59:string)
    n374 = case shown="True" w53 {
      selector: w53 -> [w82 w83]
      tunnel: [w82 w83] -> w43
      frame False {
      }
      frame True {
        n375 = local write "Apply"(FALSE ("Apply")) -> ()
      }
    }
    n376 = local read "Proper VI No"() -> (w51:i32)
    n377 = Bundle("Load Test"="Load Test", "I_Channel0"="I_Channel0", "O_Channel0"="O_Channel0", "I_Channel1"="I_Channel1", "Config P2"="Config P2", "Config R3"="Config R3", "Config R4"="Config R4", "Config R5"="Config R5", "Config R6"="Config R6", "Config R7"="Config R7", "Config P7"="Config P7", "Config R8"="Config R8", "Config P8"="Config P8", "Config R9"="Config R9", "Config P9"="Config P9", "Config R10"="Config R10", "Config P10"="Config P10", "Add Lib"="Add Lib", "OK"="OK", "Cancel"="Cancel") -> (w62:T16)  [unwired: 1 out]
    n378 = Cluster To Array(cluster=w62) -> (array=w80:bool[])
    n379 = Search 1D Array(1D array=w80, element=TRUE) -> (index of element=w79:i32)  [unwired: 1 in]
    n380 = case shown="17" w79 {
      tunnel: w59 -> [_ _ _ _ _ w434 w468 w501 w535 w571 _ _ _]
      tunnel: w58 -> [_ w199 w344 w369 w414 w433 w467 w500 w534 w570 w602 w633 _]
      tunnel: w56 -> [_ _ _ w373 _ _ _ _ _ _ _ _ _]
      tunnel: w57 -> [_ _ _ _ _ w431 w465 w498 w533 w568 _ _ _]
      tunnel: w52 -> [_ _ _ _ _ _ _ w497 _ _ _ _ _]
      tunnel: w51 -> [_ _ _ _ _ _ w463 w496 w531 w566 _ _ w666]
      tunnel: w50 -> [_ _ _ _ _ _ w464 _ w532 w567 _ _ _]
      tunnel: w46 -> [_ _ _ _ _ _ _ _ _ _ w603 w634 _]
      tunnel: w45 -> [_ w193 _ _ _ _ _ _ _ _ _ _ _]
      frame Default {
      }
      frame 0 {
        # "Load Test"
        n381 = call "CRYUnflatten Calibration 2D.vi"("Flattened Calibration"=w199) -> ("Calibration Step Out"=w198:T17)  [unwired: 8 in, 2 out]
        n382 = call "CRYGet Calibrated Device Name.vi"("Calibration"=w198) -> ("I_Signal Type Out"=w197:string[], "O_Signal Type Out"=w196:string[], "I_Calibration Out"=w194:T14[], "O_Calibration Out"=w195:T14[])  [unwired: 7 in, 4 out]
        n383 = stacked-sequence {
          seq-local: [w206 _ _ _] -> [_ w225 _ _]
          tunnel: w197 -> [_ w219 w270 _]
          tunnel: w196 -> [_ _ w280 _]
          tunnel: w195 -> [_ _ w279 _]
          tunnel: w194 -> [_ _ w277 _]
          tunnel: w193 -> [w200 _ _ _]
          frame #0 {
            # "Mode numbers:\n0 - Play & Record\n1 - Record\n2 - Signal Generator\n3 - Voltmeter\n4 - Oscilloscope\n5 - Spectrum Analyzer\n6 - Real Time Analyzer\n7 - Generator & Voltmeter\n8 - Generator & Oscilloscope\n9 - Generator & Spectrum\n10 - Generator & RTA"
            n384 = call "CRYGet Current HC Steps.vi"() -> ("Hardware setup flattened Out"=w201:string)  [unwired: 10 in, 1 out]
            n385 = call "CRYUnflatten SoundCard.vi"("Flatten SoundCard"=w201) -> ("SoundCard"=w205:T18)  [unwired: 10 out]
            n386 = call "CRYGet Upper Step Data.vi"("Type In"=enum16{"Curves", "Values", "Results", "WFM"}."WFM", "No.VI"=w200) -> ("Waveform Array"=w207:T13)  [unwired: 9 out]
            n387 = Unbundle By Name(w205) -> ("Channel Array"=w204:T4[])
            n388 = for {
              tunnel: w207 -> [w210] mode=indexing
              tunnel: [w209] -> w206 mode=indexing
              n389 = Unbundle By Name(w210) -> ("Name"=w209:string)
            }
            n390 = call "CRYGet Channel Array.vi"("Channel Array"=w204) -> ("I Channel Info Out"=→"I_channel Info":T4[], "O Channel Info Out"=→"O_channel Info":T4[])  [unwired: 9 out]
            n391 = property on="WFMRing" class="Ring (strict)"("Strings []"=w206) -> ()  [unwired: 2 in, 2 out]
          }
          frame #1 {
            w212 = 0.05 ("y")
            w228 = u8 2 ("Disabled")
            n392 = local read "Acquisition"() -> (w227:T1)
            n393 = Unbundle By Name(w227) -> ("Mode"=w239:u16, "Name"=w240:string, "use ch name"=w218:bool)
            n394 = flat-sequence {
              tunnel: [w255] -> w224
              tunnel: w219 -> [w255]
              tunnel: w222 -> [w257]
              tunnel: w224 -> [w256]
              frame #0 {
                n395 = property on="Trigger Channel1" class="Ring (strict)"("Strings []"=w255) -> ()  [unwired: 2 in, 2 out]
              }
              frame #1 {
                n396 = Search 1D Array(1D array=w256, element=w257) -> (index of element=w258:i32)  [unwired: 1 in]
                n397 = property on="Trigger Channel1" class="Ring (strict)"("Val(Sgnl)"=w258) -> ()  [unwired: 2 in, 2 out]
              }
            }
            n398 = Unbundle By Name(w227) -> ("Help"=w221:string, "trig channel"=w222:string, "triggered  record"=w223:bool, "rec pad"=w215:dbl, "Record Time"=w213:dbl, "hide play"=w233:bool, "hide rec"=w234:bool, "record table"=w217:string[][], "play table"=w220:string[][])
            n399 = property on="Mode Tab" class="TabCtl (strict)"("Value"=w239) -> ()  [unwired: 2 in, 2 out]
            n400 = property on="Record Curve Name" class="Str"("Value"=w240) -> ()  [unwired: 2 in, 2 out]
            n401 = property on="Use Channel Name" class="Bool (strict)"("Value"=w218) -> ()  [unwired: 2 in, 2 out]
            n402 = property on="Mode Select" class="Ring (strict)"("Value"=w239) -> ()  [unwired: 2 in, 2 out]
            n403 = Max & Min(x=w215, y=w212) -> (max(x,y)=w214:dbl)  [unwired: 1 out]
            n404 = property on="Triger1" class="Bool (strict)"("Val(Sgnl)"=w223) -> ()  [unwired: 2 in, 2 out]
            n405 = property on="Help" class="Str"("Value"=w221) -> ()  [unwired: 2 in, 2 out]
            n406 = Max & Min(x=w212, y=w213) -> (max(x,y)=w211:dbl)  [unwired: 1 out]
            n407 = property on="Time R0" class="DigNum (strict)"("Value"=w214) -> ()  [unwired: 2 in, 2 out]
            n408 = property on="Time R1" class="DigNum (strict)"("Value"=w211) -> ()  [unwired: 2 in, 2 out]
            n409 = for {
              tunnel: w220 -> [w260] mode=indexing
              tunnel: w225 -> [w262]
              tunnel: [w259] -> w226 mode=indexing
              n410 = Index Array(array=w260, index=1) -> (element=w263:string)
              n411 = Search 1D Array(1D array=w262, element=w263) -> (index of element=w261:i32)  [unwired: 1 out]
              n412 = case shown="0, Default" w261 {
                tunnel: w260 -> [w265 w269]
                tunnel: [w265 w266] -> w259
                frame 0, Default {
                }
                frame -1 {
                  n413 = Replace Array Subset(array=w269, new element="" ("new element/subarray"), index=1) -> (w266:string[])
                }
              }
            }
            n414 = Unbundle By Name(w227) -> ("trig level"=w237:dbl, "trig offset(sec)"=w236:dbl, "trig slop"=w235:bool, "trig unit"=w230:u8, "trig timeout(sec)"=w238:dbl)
            n415 = property on="Slop1+1" class="Bool (strict)"("Val(Sgnl)"=w235) -> ()  [unwired: 2 in, 2 out]
            n416 = property on="MP0" class="MCListbox (strict)"("ItemNames"=w226) -> ()  [unwired: 2 in, 2 out]
            n417 = property on="Trigger Level1" class="DigNum (strict)"("Value"=w237) -> ()  [unwired: 2 in, 2 out]
            n418 = property on="Trigger Offset1" class="DigNum (strict)"("Value"=w236) -> ()  [unwired: 2 in, 2 out]
            n419 = property on="Time Out1" class="DigNum (strict)"("Value"=w238) -> ()  [unwired: 2 in, 2 out]
            n420 = Not Equal To 0?(x=w230) -> (x != 0?=w229:bool)
            n421 = property on="Trigger Unit1_1" class="Bool (strict)"("Val(Sgnl)"=w229) -> ()  [unwired: 2 in, 2 out]
            n422 = Unbundle By Name(w227) -> ("rec delay"=w232:dbl, "dcc units"=w231:i8)
            n423 = disable-structure shown="Disabled" {
              frame Disabled {
                n424 = property on="Trigger Channel1" class="Ring (strict)" props=["Value"]() -> ()  [unwired: 3 in, 2 out]
              }
              frame Enabled {
              }
            }
            n425 = property on="Delay R6" class="DigNum (strict)"("Value"=w232) -> ()  [unwired: 2 in, 2 out]
            n426 = property on="Delay R7" class="DigNum (strict)"("Value"=w232) -> ()  [unwired: 2 in, 2 out]
            n427 = property on="Delay R8" class="DigNum (strict)"("Value"=w232) -> ()  [unwired: 2 in, 2 out]
            n428 = property on="Delay R9" class="DigNum (strict)"("Value"=w232) -> ()  [unwired: 2 in, 2 out]
            n429 = property on="Delay R10" class="DigNum (strict)"("Value"=w232) -> ()  [unwired: 2 in, 2 out]
            n430 = property on="Hide P P2" class="Bool (strict)"("Value"=w233) -> ()  [unwired: 2 in, 2 out]
            n431 = property on="Hide P P7" class="Bool (strict)"("Value"=w233) -> ()  [unwired: 2 in, 2 out]
            n432 = property on="Hide P P8" class="Bool (strict)"("Value"=w233) -> ()  [unwired: 2 in, 2 out]
            n433 = property on="Hide P P9" class="Bool (strict)"("Value"=w233) -> ()  [unwired: 2 in, 2 out]
            n434 = property on="Hide P P10" class="Bool (strict)"("Value"=w233) -> ()  [unwired: 2 in, 2 out]
            n435 = property on="dcc unit11" class="RadioBtnsControl (strict)"("Value"=w231) -> ()  [unwired: 2 in, 2 out]
            n436 = flat-sequence {
              tunnel: w217 -> [w248]
              tunnel: [w248] -> w216
              frame #0 {
                n437 = local read "Acquisition"() -> (w253:T1)
                n438 = local read "Calibration In"() -> (w251:string)
                n439 = local read "Hardware In"() -> (w252:string)
                n440 = call "CRYGet Current TS Steps.vi"() -> ("SelectStepNumber in Tree"=w246:i32, "Steps"=w243:T8[])  [unwired: 1 in, 9 out]
                n441 = Index Array(array=w243, index=w246) -> (element=w244:T8)
                n442 = call "CRYFlatten Acquisition.vi"("Acquisition"=w253) -> ("Acquisition flattened"=w242:string)  [unwired: 10 out]
                n443 = Bundle By Name(cluster=w244, "Seq setup flattened"=w242) -> (w245:T8)
                n444 = call "CRYReplace Acquisition Curve Name.vi"("Calibration in"=w251, "Setup in"=w245, "Hardware Setup In"=w252, "Step Setup In"=w242, "No Insert CurveLib?"=TRUE, "Type In"="AddStep") -> ("Current Name Out"=w247:string[][])  [unwired: 3 in, 2 out]
                "Origin MR0" <- w247
                n445 = call "CRYGet Changed Acquisition Curve Name.vi"("Load?"=TRUE, "New Name"=w247) -> ("Changed Name Table  out"=w250:string[][])  [unwired: 9 in]
                n446 = property on="Changed Curve" class="Arr (strict)"("Value"=w250) -> ()  [unwired: 2 in, 2 out]
                n447 = property on="Old MR0" class="Arr (strict)"("Value"=w247) -> ()  [unwired: 2 in, 2 out]
              }
            }
            n448 = property on="HideP R3" class="Bool (strict)"("Value"=w234) -> ()  [unwired: 2 in, 2 out]
            n449 = property on="Hide P R4" class="Bool (strict)"("Value"=w234) -> ()  [unwired: 2 in, 2 out]
            n450 = property on="Hide P R5" class="Bool (strict)"("Value"=w234) -> ()  [unwired: 2 in, 2 out]
            n451 = property on="Hide P R6" class="Bool (strict)"("Value"=w234) -> ()  [unwired: 2 in, 2 out]
            n452 = property on="Hide P R7" class="Bool (strict)"("Value"=w234) -> ()  [unwired: 2 in, 2 out]
            n453 = property on="Hide P R8" class="Bool (strict)"("Value"=w234) -> ()  [unwired: 2 in, 2 out]
            n454 = property on="Hide P R9" class="Bool (strict)"("Value"=w234) -> ()  [unwired: 2 in, 2 out]
            n455 = property on="Hide P R10" class="Bool (strict)"("Value"=w234) -> ()  [unwired: 2 in, 2 out]
            n456 = property on="Hide P P2" class="Bool (strict)"("Disabled"=w228) -> ()  [unwired: 2 in, 2 out]
            n457 = property on="Hide P P7" class="Bool (strict)"("Disabled"=w228) -> ()  [unwired: 2 in, 2 out]
            n458 = property on="Hide P P8" class="Bool (strict)"("Disabled"=w228) -> ()  [unwired: 2 in, 2 out]
            n459 = property on="Hide P P9" class="Bool (strict)"("Disabled"=w228) -> ()  [unwired: 2 in, 2 out]
            n460 = property on="Hide P P10" class="Bool (strict)"("Disabled"=w228) -> ()  [unwired: 2 in, 2 out]
            n461 = property on="MR0" class="Tbl (strict)"("Val(Sgnl)"=w216) -> ()  [unwired: 2 in, 2 out]
          }
          frame #2 {
            w285 = T4[] []  # Channel Info
            # "Output"
            # "Input"
            # "Get Hardware Channel Infor to Selected Signal Type"
            # "????????"
            n462 = flat-sequence {
              frame #0 {
                n463 = control-ref of="Board Tab"() -> (w333:refnum<vi>)
                n464 = control-ref of="This VI"() -> (w332:refnum<vi>)
                n465 = call "CRYAlign Steps VI Center.vi"("Tab2"=w333, "Input/Output"=TRUE ("Preview"), "VIRef"=w332) -> ()  [unwired: 1 in, 8 out]
              }
              frame #1 {
                n466 = local write "Load Test"(FALSE ("Load Test")) -> ()
                n467 = property on="Board Tab" class="TabCtl (strict)"("Visible"=TRUE) -> ()  [unwired: 2 in, 2 out]
              }
            }
            n468 = local read "I_channel Info"() -> (w286:T4[])
            n469 = local read "O_channel Info"() -> (w284:T4[])
            n470 = property on="MP0" class="MCListbox (strict)"() -> ("ItemNames"=w283:string[][])  [unwired: 2 in, 2 out]
            n471 = for {
              tunnel: w286 -> [w310] mode=indexing
              tunnel: [w309] -> w276 mode=indexing
              n472 = Unbundle By Name(w310) -> ("Name"=w309:string)
            }
            n473 = for {
              tunnel: w284 -> [w288] mode=indexing
              tunnel: [w287] -> w278 mode=indexing
              n474 = Unbundle By Name(w288) -> ("Name"=w287:string)
            }
            n475 = property on="MR0" class="Tbl (strict)"() -> ("Value"=w274:string[][])  [unwired: 2 in, 2 out]
            n476 = Index Array(array=w283, index (col)=0 ("disabled index (col)")) -> (element=w281:string[])  [unwired: 1 in]
            n477 = Index Array(array=w274, index (col)=0 ("disabled index (col)")) -> (element=w273:string[])  [unwired: 1 in]
            n478 = for {
              tunnel: w281 -> [w289] mode=indexing
              tunnel: w280 -> [w297]
              shift-right: [w295] -> w272
              shift-left: w285 -> [w294]
              tunnel: w284 -> [w290]
              tunnel: w279 -> [w292]
              tunnel: w278 -> [w291]
              i -> [w293]
              n479 = Search 1D Array(1D array=w297, element=w289) -> (index of element=w296:i32)  [unwired: 1 out]
              n480 = case shown="0, Default" w296 {
                tunnel: [w299 w308] -> w295
                tunnel: w294 -> [w300 w308]
                tunnel: w293 -> [w306 _]
                tunnel: w292 -> [w307 _]
                tunnel: w291 -> [w304 _]
                tunnel: w290 -> [w303 _]
                frame 0, Default {
                  n481 = Index Array(array=w307, index=w306) -> (element=w305:T14)
                  n482 = Unbundle By Name(w305) -> ("Calibration.Cha Name"=w298:string)
                  n483 = Search 1D Array(1D array=w304, element=w298) -> (index of element=w302:i32)  [unwired: 1 out]
                  n484 = Index Array(array=w303, index=w302) -> (element=w301:T4)
                  n485 = Build Array (concatenate)(w300, w301) -> (w299:T4[])
                }
                frame -1 {
                }
              }
            }
            n486 = for {
              tunnel: w273 -> [w311] mode=indexing
              tunnel: w270 -> [w312]
              shift-right: [w316] -> w271
              shift-left: w285 -> [w317]
              tunnel: w286 -> [w314]
              tunnel: w277 -> [w315]
              tunnel: w276 -> [w313]
              i -> [w318]
              n487 = Search 1D Array(1D array=w312, element=w311) -> (index of element=w319:i32)  [unwired: 1 out]
              n488 = case shown="0, Default" w319 {
                tunnel: [w322 w330] -> w316
                tunnel: w317 -> [w323 w330]
                tunnel: w318 -> [w328 _]
                tunnel: w315 -> [w329 _]
                tunnel: w313 -> [w326 _]
                tunnel: w314 -> [w321 _]
                frame 0, Default {
                  n489 = Index Array(array=w329, index=w328) -> (element=w327:T14)
                  n490 = Unbundle By Name(w327) -> ("Calibration.Cha Name"=w320:string)
                  n491 = Search 1D Array(1D array=w326, element=w320) -> (index of element=w325:i32)  [unwired: 1 out]
                  n492 = Index Array(array=w321, index=w325) -> (element=w324:T4)
                  n493 = Build Array (concatenate)(w323, w324) -> (w322:T4[])
                }
                frame -1 {
                }
              }
            }
            n494 = local write "Selected I_channel Info"(w271) -> ()
            n495 = local write "Selected O_channel Info"(w272) -> ()
          }
          frame #3 {
            n496 = flat-sequence {
              frame #0 {
                n497 = local read "AddStep"() -> (w336:bool)
                n498 = local write "Add Lib"(w336) -> ()
              }
              frame #1 {
                n499 = local write "AddStep"(FALSE ("AddStep")) -> ()
              }
            }
          }
        }
      }
      frame 1 {
        n500 = property on="MR0" class="Tbl (strict)"() -> ("Value"=w339:string[][])  [unwired: 2 in, 2 out]
        n501 = call "CRYUnflatten Calibration 2D.vi"("Flattened Calibration"=w344) -> ("Calibration Step Out"=w343:T17)  [unwired: 8 in, 2 out]
        n502 = Index Array(array=w339, index (col)=0 ("disabled index (col)")) -> (element=w338:string[])  [unwired: 1 in]
        n503 = local read "I_channel Info"() -> (w342:T4[])
        n504 = call "CRYSelect Signal Type Dialog.vi"("Channel Info In"=w342, "Selected Signal Type In"=w338, "Mode(0ne or More)"=FALSE, "I/O Calibration In"=w343, "In/Out Signal Type"=TRUE) -> ("Calibration 2D Out"=w346:T14[], "Selected Flag"=w347:bool, "Selected Channel Info Out"=→"Selected I_channel Info":T4[])  [unwired: 3 in, 1 out]
        n505 = case shown="True" w347 {
          tunnel: w346 -> [_ w351]
          frame False {
          }
          frame True {
            n506 = property on="Record Curve Name" class="Str"() -> ("Value"=w352:string)  [unwired: 2 in, 2 out]
            n507 = for {
              tunnel: [w360] -> w350 mode=indexing
              tunnel: w352 -> [w359]
              tunnel: w351 -> [w358] mode=indexing
              n508 = Unbundle By Name(w358) -> ("Calibration.Signal Type"=w357:string)
              n509 = Bundle("Signal Type"=w357, "Value"=w359) -> (w361:cluster{"Signal Type":string, "Value":string})  [unwired: 1 out]
              n510 = Cluster To Array(cluster=w361) -> (array=w360:string[])
            }
            n511 = flat-sequence {
              tunnel: w350 -> [w353]
              tunnel: [w353] -> w349
              frame #0 {
                n512 = local read "Acquisition"() -> (w356:T1)
                n513 = Bundle By Name(cluster=w356, "record table"=w353) -> (w354:T1)
                n514 = property on="Channels Change?" class="Bool (strict)"("Value"=TRUE ("Channels Change?")) -> ()  [unwired: 2 in, 2 out]
                n515 = local write "Acquisition"(w354) -> ()
              }
            }
            n516 = property on="MR0" class="Tbl (strict)"("Val(Sgnl)"=w349) -> ()  [unwired: 2 in, 2 out]
          }
        }
      }
      frame 2 {
        # "O_Channel0"
        n517 = property on="MP0" class="MCListbox (strict)"() -> ("ItemNames"=w365:string[][])  [unwired: 2 in, 2 out]
        n518 = local read "O_channel Info"() -> (w368:T4[])
        n519 = call "CRYUnflatten Calibration 2D.vi"("Flattened Calibration"=w369) -> ("Calibration Step Out"=w370:T17)  [unwired: 8 in, 2 out]
        n520 = Index Array(array=w365, index (col)=0 ("disabled index (col)")) -> (element=w364:string[])  [unwired: 1 in]
        n521 = call "CRYSelect Signal Type Dialog.vi"("Channel Info In"=w368, "Selected Signal Type In"=w364, "Mode(0ne or More)"=FALSE, "I/O Calibration In"=w370, "In/Out Signal Type"=FALSE) -> ("Calibration 2D Out"=w363:T14[], "Selected Flag"=w362:bool, "Selected Channel Info Out"=→"Selected O_channel Info":T4[])  [unwired: 3 in, 1 out]
        n522 = case shown="True" w362 {
          tunnel: w373 -> [_ w381]
          tunnel: w364 -> [_ w378]
          tunnel: w365 -> [_ w377]
          tunnel: w363 -> [_ w375]
          frame False {
          }
          frame True {
            # "Find in Upper Step"
            n523 = call "CRYGet Equal Category.vi"("Current StepName"=w381, "Find CategoryName"="Stimulus") -> ("setup flattened Array out"=w383:T19, "Find Flag"=w374:bool)  [unwired: 8 out]
            n524 = case shown="True" w374 {
              tunnel: w383 -> [_ w388]
              tunnel: ["" w386] -> w380
              frame False {
              }
              frame True {
                n525 = Index Array(array=w388) -> (element=w389:T20)  [unwired: 1 in]
                n526 = Unbundle By Name(w389) -> ("setup flattened"=w390:string)
                n527 = call "CRYUnflatten Stimulus.vi"("Flatten Stimulus"=w390) -> ("Stimulus"=w387:T21)  [unwired: 10 out]
                n528 = Unbundle By Name(w387) -> ("CustomStimulusName"=w386:string)
              }
            }
            n529 = for {
              tunnel: w380 -> [w399]
              tunnel: [w398] -> w379 mode=indexing
              tunnel: w378 -> [w397]
              tunnel: w377 -> [w394]
              tunnel: w375 -> [w392] mode=indexing
              # "Already selected equal signal type Test"
              n530 = Unbundle By Name(w392) -> ("Calibration.Signal Type"=w391:string)
              n531 = for {
                tunnel: w397 -> [w410] mode=indexing
                tunnel: w391 -> [w409]
                tunnel: [w408] -> w396 mode=indexing
                tunnel: [w407] -> w393
                i -> [w407]
                stop <- w408 stop-if-true
                n532 = Equal?(x=w409, y=w410) -> (x = y?=w408:bool)
              }
              n533 = Or Array Elements(Boolean array=w396) -> (logical OR=w395:bool)
              n534 = case shown="True" w395 {
                tunnel: w399 -> [w402 _]
                tunnel: [w401 w404] -> w398
                tunnel: w391 -> [w400 _]
                tunnel: w394 -> [_ w405]
                tunnel: w393 -> [_ w406]
                frame False {
                  n535 = Bundle("Signal Type"=w400, "CustomStimulusName"=w402) -> (w403:T22)  [unwired: 1 out]
                  n536 = Cluster To Array(cluster=w403) -> (array=w401:string[])
                }
                frame True {
                  n537 = Index Array(array=w405, index (row)=w406) -> (element=w404:string[])  [unwired: 1 in]
                }
              }
            }
            n538 = property on="MP0" class="MCListbox (strict)"("ItemNames"=w379) -> ()  [unwired: 2 in, 2 out]
            n539 = local read "Acquisition"() -> (w384:T1)
            n540 = Bundle By Name(cluster=w384, "play table"=w379) -> (w376:T1)
            n541 = local write "Acquisition"(w376) -> ()
          }
        }
      }
      frame 3 {
        n542 = property on="MR0" class="Tbl (strict)"() -> ("Value"=w416:string[][])  [unwired: 2 in, 2 out]
        n543 = call "CRYUnflatten Calibration 2D.vi"("Flattened Calibration"=w414) -> ("Calibration Step Out"=w419:T17)  [unwired: 8 in, 2 out]
        n544 = Index Array(array=w416, index (col)=0 ("disabled index (col)")) -> (element=w415:string[])  [unwired: 1 in]
        n545 = local read "I_channel Info"() -> (w418:T4[])
        n546 = call "CRYSelect Signal Type Dialog.vi"("Channel Info In"=w418, "Selected Signal Type In"=w415, "Mode(0ne or More)"=FALSE, "I/O Calibration In"=w419, "In/Out Signal Type"=TRUE) -> ("Calibration 2D Out"=w411:T14[], "Selected Flag"=w412:bool, "Selected Channel Info Out"=w413:T4[])  [unwired: 3 in, 1 out]
        n547 = local write "Selected I_channel Info"(w413) -> ()
        n548 = case shown="True" w412 {
          tunnel: w411 -> [_ w423]
          frame False {
          }
          frame True {
            n549 = for {
              tunnel: [w428] -> w422 mode=indexing
              tunnel: w423 -> [w426] mode=indexing
              n550 = Unbundle By Name(w426) -> ("Calibration.Signal Type"=w427:string)
              n551 = property on="Record Curve Name" class="Str"() -> ("Value"=w429:string)  [unwired: 2 in, 2 out]
              n552 = Bundle("Signal Type"=w427, "Value"=w429) -> (w430:cluster{"Signal Type":string, "Value":string})  [unwired: 1 out]
              n553 = Cluster To Array(cluster=w430) -> (array=w428:string[])
            }
            n554 = local read "Acquisition"() -> (w425:T1)
            n555 = Bundle By Name(cluster=w425, "record table"=w422) -> (w424:T1)
            n556 = property on="MR0" class="Tbl (strict)"("Val(Sgnl)"=w422) -> ()  [unwired: 2 in, 2 out]
            n557 = local write "Acquisition"(w424) -> ()
          }
        }
      }
      frame 4, 10, 12, 14, 16 {
        # "Signal Generator"
        n558 = flat-sequence {
          tunnel: [w439] -> w432
          tunnel: w432 -> [w452]
          tunnel: w433 -> [w449]
          tunnel: w434 -> [w450]
          tunnel: w431 -> [w446]
          frame #0 {
            n559 = local read "Acquisition"() -> (w439:T1)
            n560 = Unbundle By Name(w439) -> ("sine gen setting"=w438:string)
            n561 = call "CRYUnflatten Signal Generator.vi"("Flat Signal Gen'r settings"=w438) -> ("Signal Gen'r settings"=w437:T23)  [unwired: 10 out]
            n562 = global write "CRYMisc vis settings global.vi" "Signal Gen'r settings"(w437) -> ()
            n563 = property on="Board Tab" class="TabCtl (strict)"("Disabled"=u8 2) -> ()  [unwired: 2 in, 2 out]
            n564 = global write "CRYMisc vis settings global.vi" "Menu?"(FALSE ("Menu?")) -> ()
          }
          frame #1 {
            n565 = call "CRYSignal Generator.vi"("Manual"=FALSE, "Execution control"=w446, "Mute"=TRUE, "Hardware in"=w450, "Calibration in"=w449) -> ("Sigal generator setup Out"=w451:string)  [unwired: 5 in, 5 out]
            n566 = call "CRYUnflatten Signal Generator.vi"("Flat Signal Gen'r settings"=w451) -> ("Signal Gen'r settings"=w444:T23)  [unwired: 10 out]
            n567 = Unbundle By Name(w444) -> ("gen'r mode"=w442:i32, "wav play mode"=w445:i32, "Play Sine Wave"=w441:i32)
            n568 = case shown="0" w442 {
              tunnel: w445 -> [_ w458]
              tunnel: [w453 w457] -> w443
              tunnel: w441 -> [w454 _]
              frame 0 {
                n569 = case shown="1" w454 {
                  tunnel: [u8 2 ("Disabled") u8 0 ("Disabled")] -> w453
                  frame 0, Default {
                  }
                  frame 1 {
                  }
                }
              }
              frame 1, Default {
                n570 = case shown="2" w458 {
                  tunnel: [u8 2 ("Disabled") u8 0 ("Disabled") u8 0 ("Disabled")] -> w457
                  frame 0, Default {
                  }
                  frame 1 {
                  }
                  frame 2 {
                  }
                }
              }
            }
            n571 = property on="Hide P P2" class="Bool (strict)"("Disabled"=w443) -> ()  [unwired: 2 in, 2 out]
            n572 = property on="Hide P P7" class="Bool (strict)"("Disabled"=w443) -> ()  [unwired: 2 in, 2 out]
            n573 = property on="Hide P P8" class="Bool (strict)"("Disabled"=w443) -> ()  [unwired: 2 in, 2 out]
            n574 = property on="Hide P P9" class="Bool (strict)"("Disabled"=w443) -> ()  [unwired: 2 in, 2 out]
            n575 = property on="Hide P P10" class="Bool (strict)"("Disabled"=w443) -> ()  [unwired: 2 in, 2 out]
            n576 = Bundle By Name(cluster=w452, "sine gen setting"=w451) -> (w440:T1)
            n577 = local write "Acquisition"(w440) -> ()
          }
          frame #2 {
            n578 = property on="Board Tab" class="TabCtl (strict)"("Disabled"=u8 0) -> ()  [unwired: 2 in, 2 out]
          }
        }
      }
      frame 5, 9 {
        # "Multimetor"
        n579 = flat-sequence {
          tunnel: [w471] -> w466
          tunnel: w465 -> [w478]
          tunnel: w468 -> [w477]
          tunnel: w467 -> [w476]
          tunnel: w466 -> [w481]
          tunnel: w464 -> [w475]
          tunnel: w463 -> [w474]
          frame #0 {
            n580 = local read "Acquisition"() -> (w471:T1)
            n581 = Unbundle By Name(w471) -> ("voltmeter setting"=w473:string)
            n582 = call "CRYUnflatten Multimeter.vi"("Flat Voltmeter setup"=w473) -> ("Voltmeter Settings"=w472:T24)  [unwired: 10 out]
            n583 = global write "CRYMisc vis settings global.vi" "Voltmeter Settings"(w472) -> ()
            n584 = property on="Board Tab" class="TabCtl (strict)"("Disabled"=u8 2) -> ()  [unwired: 2 in, 2 out]
            n585 = global write "CRYMisc vis settings global.vi" "Menu?"(FALSE ("Menu?")) -> ()
          }
          frame #1 {
            n586 = call "CRYMultimeter.vi"("Calibration in"=w476, "Hardware in"=w477, "Manual"=FALSE, "Execution control"=w478) -> ("Canceled?"=w479:bool)  [unwired: 7 in, 8 out]
            n587 = case shown="False" w479 {
              tunnel: w481 -> [w492 _]
              tunnel: w475 -> [_ _]
              tunnel: w474 -> [_ _]
              frame False {
                n588 = global read "CRYMisc vis settings global.vi" "Voltmeter Settings"() -> (w489:T24)
                n589 = Unbundle By Name(w489) -> ("lin/exp avg"=w490:u16, "Signal Type"=w484:string)
                n590 = property on="MR0" class="Tbl (strict)"() -> ("Value"=w487:string[][])  [unwired: 2 in, 2 out]
                n591 = Index Array(array=w487) -> (element=w486:string[])  [unwired: 2 in]
                n592 = Replace Array Subset(array=w486, new element=w484) -> (w485:string[])  [unwired: 1 in]
                n593 = call "CRYFlatten Multimeter.vi"("Voltmeter Settings"=w489) -> ("Flat Voltmeter setup"=w491:string)  [unwired: 10 out]
                n594 = Build Array(w485) -> (w483:string[][])
                n595 = property on="MR0" class="Tbl (strict)"("Val(Sgnl)"=w483) -> ()  [unwired: 2 in, 2 out]
                n596 = Bundle By Name(cluster=w492, "voltmeter setting"=w491, "record table"=w483) -> (w482:T1)
                n597 = case shown="1" w490 {
                  tunnel: [u8 0 ("Disabled") u8 2 ("Disabled")] -> w488
                  frame 0, Default {
                  }
                  frame 1 {
                  }
                }
                n598 = local write "Acquisition"(w482) -> ()
                n599 = property on="HideP R3" class="Bool (strict)"("Disabled"=w488) -> ()  [unwired: 2 in, 2 out]
                n600 = property on="Hide P R7" class="Bool (strict)"("Disabled"=w488) -> ()  [unwired: 2 in, 2 out]
              }
              frame True {
              }
            }
          }
          frame #2 {
            n601 = property on="Board Tab" class="TabCtl (strict)"("Disabled"=u8 0) -> ()  [unwired: 2 in, 2 out]
          }
        }
      }
      frame 6, 11 {
        n602 = flat-sequence {
          tunnel: [w504] -> w499
          tunnel: w499 -> [w509]
          tunnel: w500 -> [w512]
          tunnel: w501 -> [w513]
          tunnel: w498 -> [w510]
          tunnel: w497 -> [w508]
          tunnel: w496 -> [w507]
          frame #0 {
            n603 = local read "Acquisition"() -> (w504:T1)
            n604 = Unbundle By Name(w504) -> ("scope_fft setting"=w506:string)
            n605 = call "CRYUnflatten Scope-FFT.vi"("Flat Scope-FFT setup"=w506) -> ("Scope-FFT settings"=w505:T25)  [unwired: 10 out]
            n606 = global write "CRYMisc vis settings global.vi" "Scope-FFT settings"(w505) -> ()
            n607 = global write "CRYMisc vis settings global.vi" "Menu?"(FALSE ("Menu?")) -> ()
            n608 = property on="Board Tab" class="TabCtl (strict)"("Disabled"=u8 2) -> ()  [unwired: 2 in, 2 out]
          }
          frame #1 {
            w515 = u32 0 items=["Time", "Spectrum"] ("Mode")
            n609 = call "CRYScope-FFT.vi"("Mode"=w515, "Hardware"=w513, "Execution control"=w510, "Manual"=FALSE, "Calibration"=w512) -> ("scope-fft setup Out"=w516:string, "Canceled"=w511:bool)  [unwired: 7 in, 6 out]
            n610 = case shown="False" w511 {
              tunnel: w509 -> [w520 _]
              tunnel: w516 -> [w525 _]
              tunnel: w508 -> [_ _]
              tunnel: w507 -> [_ _]
              frame False {
                n611 = call "CRYUnflatten Scope-FFT.vi"("Flat Scope-FFT setup"=w525) -> ("Scope-FFT settings"=w524:T25)  [unwired: 10 out]
                n612 = property on="MR0" class="Tbl (strict)"() -> ("Value"=w523:string[][])  [unwired: 2 in, 2 out]
                n613 = Unbundle By Name(w524) -> ("lin/exp avg"=w527:i32, "Signal Type"=w519:string)
                n614 = Index Array(array=w523) -> (element=w522:string[])  [unwired: 2 in]
                n615 = Replace Array Subset(array=w522, new element=w519) -> (w521:string[])  [unwired: 1 in]
                n616 = Build Array(w521) -> (w518:string[][])
                n617 = Bundle By Name(cluster=w520, "scope_fft setting"=w525, "record table"=w518) -> (w517:T1)
                n618 = property on="MR0" class="Tbl (strict)"("Val(Sgnl)"=w518) -> ()  [unwired: 2 in, 2 out]
                n619 = local write "Acquisition"(w517) -> ()
                n620 = case shown="1" w527 {
                  tunnel: [u8 0 ("Disabled") u8 2 ("Disabled")] -> w526
                  frame 0, Default {
                  }
                  frame 1 {
                  }
                }
                n621 = property on="Hide P R4" class="Bool (strict)"("Disabled"=w526) -> ()  [unwired: 2 in, 2 out]
                n622 = property on="Hide P R8" class="Bool (strict)"("Disabled"=w526) -> ()  [unwired: 2 in, 2 out]
              }
              frame True {
              }
            }
          }
          frame #2 {
            n623 = property on="Board Tab" class="TabCtl (strict)"("Disabled"=u8 0) -> ()  [unwired: 2 in, 2 out]
          }
        }
      }
      frame 7, 13 {
        n624 = flat-sequence {
          tunnel: [w539] -> w536
          tunnel: w533 -> [w544]
          tunnel: w535 -> [w547]
          tunnel: w534 -> [w546]
          tunnel: w536 -> [w551]
          tunnel: w532 -> [w543]
          tunnel: w531 -> [w542]
          frame #0 {
            n625 = local read "Acquisition"() -> (w539:T1)
            n626 = Unbundle By Name(w539) -> ("scope_fft setting"=w541:string)
            n627 = call "CRYUnflatten Scope-FFT.vi"("Flat Scope-FFT setup"=w541) -> ("Scope-FFT settings"=w540:T25)  [unwired: 10 out]
            n628 = global write "CRYMisc vis settings global.vi" "Scope-FFT settings"(w540) -> ()
            n629 = property on="Board Tab" class="TabCtl (strict)"("Disabled"=u8 2) -> ()  [unwired: 2 in, 2 out]
            n630 = global write "CRYMisc vis settings global.vi" "Menu?"(FALSE ("Menu?")) -> ()
          }
          frame #1 {
            w549 = u32 1 items=["Time", "Spectrum"] ("Mode")
            n631 = call "CRYScope-FFT.vi"("Mode"=w549, "Hardware"=w547, "Execution control"=w544, "Manual"=FALSE, "Calibration"=w546) -> ("scope-fft setup Out"=w550:string, "Canceled"=w545:bool)  [unwired: 7 in, 6 out]
            n632 = case shown="False" w545 {
              tunnel: w551 -> [w561 _]
              tunnel: w550 -> [w559 _]
              tunnel: w543 -> [_ _]
              tunnel: w542 -> [_ _]
              frame False {
                n633 = call "CRYUnflatten Scope-FFT.vi"("Flat Scope-FFT setup"=w559) -> ("Scope-FFT settings"=w558:T25)  [unwired: 10 out]
                n634 = Unbundle By Name(w558) -> ("lin/exp avg"=w562:i32, "Signal Type"=w554:string)
                n635 = property on="MR0" class="Tbl (strict)"() -> ("Value"=w557:string[][])  [unwired: 2 in, 2 out]
                n636 = Index Array(array=w557) -> (element=w556:string[])  [unwired: 2 in]
                n637 = case shown="1" w562 {
                  tunnel: [u8 0 ("Disabled") u8 2 ("Disabled")] -> w560
                  frame 0, Default {
                  }
                  frame 1 {
                  }
                }
                n638 = Replace Array Subset(array=w556, new element=w554) -> (w555:string[])  [unwired: 1 in]
                n639 = Build Array(w555) -> (w553:string[][])
                n640 = Bundle By Name(cluster=w561, "scope_fft setting"=w559, "record table"=w553) -> (w552:T1)
                n641 = property on="Hide P R5" class="Bool (strict)"("Disabled"=w560) -> ()  [unwired: 2 in, 2 out]
                n642 = property on="Hide P R9" class="Bool (strict)"("Disabled"=w560) -> ()  [unwired: 2 in, 2 out]
                n643 = property on="MR0" class="Tbl (strict)"("Val(Sgnl)"=w553) -> ()  [unwired: 2 in, 2 out]
                n644 = local write "Acquisition"(w552) -> ()
              }
              frame True {
              }
            }
          }
          frame #2 {
            n645 = property on="Board Tab" class="TabCtl (strict)"("Disabled"=u8 0) -> ()  [unwired: 2 in, 2 out]
          }
        }
      }
      frame 8, 15 {
        n646 = flat-sequence {
          tunnel: [w574] -> w569
          tunnel: w568 -> [w579]
          tunnel: w571 -> [w582]
          tunnel: w570 -> [w581]
          tunnel: w569 -> [w584]
          tunnel: w567 -> [w578]
          tunnel: w566 -> [w577]
          frame #0 {
            n647 = local read "Acquisition"() -> (w574:T1)
            n648 = Unbundle By Name(w574) -> ("rta setting"=w576:string)
            n649 = call "CRYUnflatten RTA.vi"("Flat RTA setup"=w576) -> ("RTA settings"=w575:T26)  [unwired: 10 out]
            n650 = global write "CRYMisc vis settings global.vi" "Menu?"(FALSE ("Menu?")) -> ()
            n651 = property on="Board Tab" class="TabCtl (strict)"("Disabled"=u8 2) -> ()  [unwired: 2 in, 2 out]
            n652 = global write "CRYMisc vis settings global.vi" "RTA settings"(w575) -> ()
          }
          frame #1 {
            n653 = call "CRYRTA.vi"("Manual"=FALSE, "Hardware in"=w582, "Execution control"=w579, "Calibration in"=w581) -> ("Canceled?"=w580:bool)  [unwired: 5 in, 6 out]
            n654 = case shown="False" w580 {
              tunnel: w584 -> [w591 _]
              tunnel: w578 -> [_ _]
              tunnel: w577 -> [_ _]
              frame False {
                n655 = global read "CRYMisc vis settings global.vi" "RTA settings"() -> (w593:T27)
                n656 = Unbundle By Name(w593) -> ("lin/exp"=w595:i32, "Signal Type"=w587:string)
                n657 = property on="MR0" class="Tbl (strict)"() -> ("Value"=w590:string[][])  [unwired: 2 in, 2 out]
                n658 = call "CRYFlatten RTA.vi"("RTA settings"=w593) -> ("Flat RTA settings"=w592:string)  [unwired: 10 out]
                n659 = Index Array(array=w590) -> (element=w589:string[])  [unwired: 2 in]
                n660 = case shown="0, Default" w595 {
                  tunnel: [u8 0 ("Disabled") u8 2 ("Disabled")] -> w594
                  frame 0, Default {
                  }
                  frame 1 {
                  }
                }
                n661 = Replace Array Subset(array=w589, new element=w587) -> (w588:string[])  [unwired: 1 in]
                n662 = Build Array(w588) -> (w586:string[][])
                n663 = Bundle By Name(cluster=w591, "rta setting"=w592, "record table"=w586) -> (w585:T1)
                n664 = property on="Hide P R10" class="Bool (strict)"("Disabled"=w594) -> ()  [unwired: 2 in, 2 out]
                n665 = property on="Hide P R6" class="Bool (strict)"("Disabled"=w594) -> ()  [unwired: 2 in, 2 out]
                n666 = property on="MR0" class="Tbl (strict)"("Val(Sgnl)"=w586) -> ()  [unwired: 2 in, 2 out]
                n667 = local write "Acquisition"(w585) -> ()
              }
              frame True {
              }
            }
          }
          frame #2 {
            n668 = property on="Board Tab" class="TabCtl (strict)"("Disabled"=u8 0) -> ()  [unwired: 2 in, 2 out]
          }
        }
      }
      frame 17 {
        n669 = local read "Acquisition"() -> (w604:T1)
        n670 = flat-sequence {
          tunnel: w604 -> [w616]
          tunnel: [w614] -> w611
          tunnel: [w616] -> w610
          tunnel: [w612] -> w599
          tunnel: [w625] -> w609
          tunnel: w603 -> [w620]
          tunnel: [w622] -> w608
          tunnel: w611 -> [w625]
          tunnel: w610 -> [w623]
          tunnel: w607 -> [w619]
          tunnel: w602 -> [w618]
          tunnel: [w617] -> w600
          tunnel: w599 -> [w617]
          tunnel: w609 -> [_]
          tunnel: w608 -> [_]
          tunnel: [w626] -> w601
          tunnel: w600 -> [w626]
          tunnel: w601 -> [w627]
          frame #0 {
            n671 = local read "Proper VI No"() -> (w612:i32)
            n672 = Build Array(w612) -> (w615:i32[])
            n673 = call "CRYGet Curve Library Data Name.vi"("nData"=w615, "sAction"="GetNamebyStep" ("sOption")) -> ("sNames"=w614:string[])  [unwired: 6 in, 3 out]
          }
          frame #1 {
            n674 = call "CRYFlatten Acquisition.vi"("Acquisition"=w623) -> ("Acquisition flattened"=w624:string)  [unwired: 10 out]
            n675 = call "CRYReplace Acquisition Curve Name.vi"("Calibration in"=w618, "Setup in"=w619, "Hardware Setup In"=w620, "Step Setup In"=w624, "Type In"="AddStep") -> ("Inserted Names Out"=w622:string[])  [unwired: 4 in, 2 out]
          }
          frame #2 {
            n676 = call "CRYChange Name by Step Editor.vi"() -> ()  [unwired: 12 in]
          }
          frame #3 {
            n677 = global read "CRYStepSetup Global.vi" "Load from AddStep"() -> (w628:bool)
            n678 = case shown="True" w628 {
              tunnel: w627 -> [_ w631]
              frame False {
              }
              frame True {
                n679 = global write "CRYStepSetup Global.vi" "Load from AddStep"(FALSE ("Load from AddStep")) -> ()
                n680 = call "CRYStepData Manipulate.vi"("sAction"="Backup", "StepNo."=w631) -> ()  [unwired: 10 in]
              }
            }
            n681 = local write "Add Lib"(FALSE ("Add Lib")) -> ()
          }
        }
        n682 = call "CRYGet Current TS Steps.vi"() -> ("SelectStepNumber in Tree"=w605:i32, "Steps"=w606:T8[])  [unwired: 1 in, 9 out]
        n683 = Index Array(array=w606, index=w605) -> (element=w607:T8)
      }
      frame 18 {
        n684 = flat-sequence {
          tunnel: w634 -> [w638]
          tunnel: w633 -> [w637]
          frame #0 {
            n685 = global read "CRYMainGlobal.vi" "Access Level"() -> (w636:enum16{"Engineer", "Technician", "Operator"})
            n686 = case shown="\"Technician\", Default" w636 {
              tunnel: w638 -> [w640 _]
              tunnel: w637 -> [w639 _]
              frame "Engineer" {
                n687 = flat-sequence {
                  tunnel: [w649] -> w642
                  tunnel: [w643] -> w641
                  tunnel: w639 -> [w656]
                  tunnel: w642 -> [_]
                  tunnel: w640 -> [w657]
                  tunnel: w641 -> [w653]
                  frame #0 {
                    n688 = local read "Proper VI No"() -> (w646:i32)
                    n689 = local read "Acquisition"() -> (w647:T1)
                    n690 = local read "Proper VI No"() -> (w651:i32)
                    n691 = call "CRYFlatten Acquisition.vi"("Acquisition"=w647) -> ("Acquisition flattened"=w643:string)  [unwired: 10 out]
                    n692 = Build Array(w651) -> (w650:i32[])
                    n693 = call "CRYPreUpdate Sequence.vi"("EventName"="SequenceUpdate", "Proper VI No"=w646, "Step flattened Arg2"=w643, "AllChangeFlg"=TRUE ("Name/Identifier")) -> ()  [unwired: 12 in]
                    n694 = call "CRYGet Curve Library Data Name.vi"("nData"=w650, "sAction"="GetNamebyStep" ("sOption")) -> ("sNames"=w649:string[])  [unwired: 6 in, 3 out]
                  }
                  frame #1 {
                    n695 = call "CRYGet Current TS Steps.vi"() -> ("SelectStepNumber in Tree"=w652:i32, "Steps"=w655:T8[])  [unwired: 1 in, 9 out]
                    n696 = Index Array(array=w655, index=w652) -> (element=w654:T8)
                    n697 = call "CRYReplace Acquisition Curve Name.vi"("Calibration in"=w656, "Setup in"=w654, "Hardware Setup In"=w657, "Step Setup In"=w653, "Type In"="StepOK") -> ()  [unwired: 4 in, 3 out]
                  }
                  frame #2 {
                    n698 = call "CRYChange Name by Step Editor.vi"() -> ()  [unwired: 12 in]
                  }
                }
              }
              frame "Technician", Default {
                n699 = call "CRYGet Error Message.vi"("Kind"="Step Setup") -> ("Window Title"=w661:string)  [unwired: 5 in, 5 out]
                n700 = call "CRYGet Access Level Message.vi"("sAction"="OK") -> ("Multibyte string"=w663:string)  [unwired: 10 in]
                n701 = call "CRYMessage Dialog.vi"("Window Title"=w661, "YesNoCancel"=T9."OK", "Message Content"=w663) -> ()  [unwired: 7 in, 2 out]
              }
            }
          }
          frame #1 {
            n702 = local write "OK"(FALSE ("OK")) -> ()
          }
        }
        n703 = local write "stop"(TRUE ("stop")) -> ()
      }
      frame 19 {
        n704 = flat-sequence {
          tunnel: w666 -> [w667]
          frame #0 {
            n705 = call "CRYStepData Manipulate.vi"("sAction"="Restore", "StepNo."=w667) -> ()  [unwired: 10 in]
          }
          frame #1 {
            n706 = local write "Cancel"(FALSE ("Cancel")) -> ()
          }
        }
        n707 = local write "stop"(TRUE ("stop")) -> ()
      }
    }
    n708 = case shown="True" "Apply" {
      tunnel: w56 -> [_ w86]
      frame False {
      }
      frame True {
        n709 = global read "CRYMainGlobal.vi" "Access Level"() -> (w85:enum16{"Engineer", "Technician", "Operator"})
        n710 = case shown="\"Engineer\"" w85 {
          tunnel: w86 -> [w100 _]
          frame "Engineer" {
            n711 = local read "Selected O_channel Info"() -> (w98:T4[])
            n712 = local read "Selected O_channel Info"() -> (w89:T4[])
            n713 = local read "Selected I_channel Info"() -> (w99:T4[])
            n714 = local read "Selected I_channel Info"() -> (w90:T4[])
            n715 = local read "Time R0"() -> (w96:dbl)
            n716 = local read "Time R1"() -> (w94:dbl)
            n717 = property on="Mode Select" class="Ring (strict)"() -> ("Value"=w92:u16)  [unwired: 2 in, 2 out]
            n718 = property on="Record Curve Name" class="Str"() -> ("Value"=w93:string)  [unwired: 2 in, 2 out]
            n719 = call "CRYCheck Input Parameter.vi"("Record Curve Name"=w93, "Numeric"=w92, "Record Time"=w94, "Padding Time"=w96) -> ("Run flag"=w95:bool)  [unwired: 7 in]
            n720 = call "CRYCheck Channel Repeat.vi"("Selected channel Info"=w98) -> ("Run flag"=w97:bool)  [unwired: 10 out]
            n721 = call "CRYCheck Channel Repeat.vi"("Selected channel Info"=w99) -> ("Run flag"=w91:bool)  [unwired: 10 out]
            n722 = call "CRYCheck Open Two Asio Driver.vi"("Selected channel Info"=w90) -> ("Run flag"=w87:bool)  [unwired: 10 in]
            n723 = call "CRYCheck Open Two Asio Driver.vi"("Selected channel Info"=w89) -> ("Run flag"=w88:bool)  [unwired: 10 in]
            n724 = Compound Arithmetic op=AND(w95, w91, w97, w87, w88) -> (w101:bool)
            n725 = case shown="True" w101 {
              tunnel: w100 -> [_ w144]
              tunnel: w95 -> [w110 _]
              tunnel: w92 -> [w109 _]
              tunnel: w88 -> [w107 _]
              tunnel: w87 -> [w108 _]
              frame False {
                w105 = FALSE ("Apply")
                n726 = And(x=w108, y=w107) -> (x .and. y?=w102:bool)
                n727 = case shown="Default" w109 {
                  tunnel: w110 -> [_ w118]
                  tunnel: [w112 w117] -> w104
                  tunnel: [w111 w116] -> w103
                  tunnel: w102 -> [_ w115]
                  frame 11 {
                    n728 = call "CRYGet Error Message.vi"("Error No"=7, "Kind"="Acquisition") -> ("Message"=w111:string, "Window Title"=w112:string)  [unwired: 4 in, 4 out]
                  }
                  frame Default {
                    n729 = case shown="True" w118 {
                      tunnel: [w120 w125] -> w117
                      tunnel: [w119 w124] -> w116
                      tunnel: w115 -> [_ w123]
                      frame False {
                        n730 = call "CRYGet Error Message.vi"("Error No"=6, "Kind"="Acquisition") -> ("Message"=w119:string, "Window Title"=w120:string)  [unwired: 4 in, 4 out]
                      }
                      frame True {
                        n731 = case shown="False" w123 {
                          tunnel: [w127 w131] -> w125
                          tunnel: [w126 w130] -> w124
                          frame True {
                            n732 = call "CRYGet Error Message.vi"("Error No"=5, "Kind"="Acquisition") -> ("Message"=w126:string, "Window Title"=w127:string)  [unwired: 4 in, 4 out]
                          }
                          frame False {
                            n733 = call "CRYGet Error Message.vi"("Error No"=9, "Kind"="Acquisition") -> ("Message"=w130:string, "Window Title"=w131:string)  [unwired: 4 in, 4 out]
                          }
                        }
                      }
                    }
                  }
                }
                n734 = global write "CRYMainGlobal.vi" "Acq Stop"(FALSE ("Acquisition Stop")) -> ()
                n735 = local write "Started"(w105) -> ()
                n736 = local write "Apply"(w105) -> ()
                n737 = call "CRYMessage Dialog.vi"("Window Title"=w104, "Message Content"=w103) -> ()  [unwired: 8 in, 2 out]
              }
              frame True {
                n738 = flat-sequence {
                  tunnel: [w150] -> w142
                  tunnel: [w146] -> w139
                  tunnel: [w145] -> w135
                  tunnel: [w157] -> w143
                  tunnel: w142 -> [w158]
                  tunnel: [w156] -> w140
                  tunnel: w139 -> [w156]
                  tunnel: [w152] -> w136
                  tunnel: w135 -> [w152]
                  tunnel: w144 -> [w182]
                  tunnel: w143 -> [w181]
                  tunnel: [w180] -> w141
                  tunnel: w140 -> [w180]
                  tunnel: [w179] -> w138
                  tunnel: [w176] -> w137
                  tunnel: w136 -> [w176]
                  tunnel: [w175] -> w134
                  tunnel: w141 -> [w185]
                  tunnel: w138 -> [w186]
                  tunnel: w137 -> [w184]
                  tunnel: w134 -> [w183]
                  frame #0 {
                    n739 = local read "Proper VI No"() -> (w147:i32)
                    n740 = local read "Acquisition"() -> (w151:T1)
                    n741 = call "CRYFlatten Acquisition.vi"("Acquisition"=w151) -> ("Acquisition flattened"=w150:string)  [unwired: 10 out]
                    n742 = Build Array(w147) -> (w148:i32[])
                    n743 = call "CRYGet Curve Library Data Name.vi"("nData"=w148, "sAction"="GetNamebyStep" ("sOption")) -> ("sNames"=w146:string[], "Type Out"=w145:string[])  [unwired: 6 in, 2 out]
                  }
                  frame #1 {
                    n744 = call "CRYGet Current TS Steps.vi"() -> ("SelectStepNumber in Tree"=w159:i32, "Steps"=w160:T8[])  [unwired: 1 in, 9 out]
                    n745 = local write "Started"(TRUE ("Started")) -> ()
                    n746 = global write "CRYMainGlobal.vi" "Acq Stop"(FALSE ("Acquisition Stop")) -> ()
                    n747 = Index Array(array=w160, index=w159) -> (element=w153:T8)
                    n748 = Bundle By Name(cluster=w153, "Seq setup flattened"=w158) -> (w157:T8)
                    n749 = property on="Mode Select" class="Ring (strict)"() -> ("Value"=w154:u16)  [unwired: 2 in, 2 out]
                    n750 = case shown="0, Default" w154 {
                      tunnel: [w166 string[][] []] -> w155
                      frame 0, Default {
                        n751 = property on="Changed Curve" class="Arr (strict)"() -> ("Value"=w173:string[][])  [unwired: 2 in, 2 out]
                        n752 = Index Array(array=w173, index (col) #1=1 ("index"), index (col) #2=2 ("index"), index (col) #3=3 ("index"), index (col) #4=4 ("index")) -> (element #1=w170:string[], element #2=w165:string[], element #3=w171:string[], element #4=w163:string[])  [unwired: 4 in]
                        n753 = Build Array(w170, w165, w171, w163) -> (w172:string[][])
                        n754 = Transpose 2D Array(2D array=w172) -> (transposed array=w166:string[][])
                      }
                      frame 2 {
                      }
                    }
                    n755 = global write "CRYMainGlobal.vi" "Changed Curve State"(w155) -> ()
                  }
                  frame #2 {
                    n756 = local read "Calibration In"() -> (w177:string)
                    n757 = local read "Hardware In"() -> (w178:string)
                    n758 = call "CRYAcquisition.vi"("Setup in"=w181, "Step name"=w182, "Hardware in"=w178, "Calibration in"=w177) -> ("Types Out"=w175:string[], "Inserted Names Out"=w179:string[])  [unwired: 3 in, 7 out]
                  }
                  frame #3 {
                    w187 = FALSE ("Apply")
                    n759 = call "CRYChange Name by Step Editor.vi"("New Names Type"=w183, "Old Names Type"=w184, "Old Names"=w185, "New Names"=w186) -> ()  [unwired: 8 in]
                    n760 = global write "CRYMainGlobal.vi" "Acq Stop"(FALSE ("Acquisition Stop")) -> ()
                    n761 = local write "Started"(w187) -> ()
                    n762 = local write "Apply"(w187) -> ()
                  }
                }
              }
            }
          }
          frame "Operator", Default {
            n763 = call "CRYGet Error Message.vi"("Kind"="Step Setup") -> ("Window Title"=w191:string)  [unwired: 5 in, 5 out]
            n764 = call "CRYGet Access Level Message.vi"() -> ("Multibyte string"=w189:string)  [unwired: 11 in]
            n765 = call "CRYMessage Dialog.vi"("Window Title"=w191, "YesNoCancel"=T9."OK", "Message Content"=w189) -> ()  [unwired: 7 in, 2 out]
          }
        }
      }
    }
  }
  n766 = flat-sequence {
    tunnel: w1 -> [_]
    frame #0 {
      n767 = control-ref of="This VI"() -> (w963:refnum<vi>)
      n768 = call "CRYWork Before Step Close.vi"("StepVI Ref"=w963) -> ()  [unwired: 11 in]
    }
    frame #1 {
      n769 = local write "EndFlag"(TRUE ("EndFlag")) -> ()
    }
  }
